vi "Experiment Python Control.vi"() -> ()   [LabVIEW 2015]
uses:
  <vilib>/Platform/TimedLoop/XDataNode/timing_clust.ctl
  <vilib>/Platform/TimedLoop/XDataNode/nitl_modes.ctl
  <vilib>/Platform/TimedLoop/XDataNode/wakeup.ctl
  <vilib>/DAQmx/read.llb/DAQmx Read (Analog 1D DBL NChan 1Samp).vi
  <vilib>/DAQmx/create/channels.llb/DAQmx Create Channel (AI-Voltage-Basic).vi
  <vilib>/Enthought/Python Integration Toolkit/api/Unpack Double.vi
  <vilib>/DAQmx/miscellaneous.llb/DAQmx Fill In Error Info.vi
  <vilib>/Platform/TimedLoop/XDataNode/XDataNode.xnode
  Program Files/neMESYS_SDK/neMESYS LabVIEW Kit/neMESYS LabVIEW Integration Kit.lvlib
  <vilib>/Platform/TimedLoop/XDataNode/XDNodeRunTimeDep.lvlib
  Conor/Temp CN7500/Omega CN7500/Omega CN7500.lvlib
  <vilib>/Enthought/Python Integration Toolkit/Python Integration Toolkit.lvlib
panel:
  out "Desired Conc Not Possible":bool
  out "Boolean 7":bool
  out "Boolean 6":bool
  out "Boolean 5":bool
  out "Boolean 4":bool
  out "Boolean 3":bool
  out "Boolean 2":bool
  out "Boolean 1":bool
  out "Boolean 8":bool
  out "Boolean 0":bool
  out "Flow 8":dbl
  out "Conc 8":dbl
  out "Temp 8":dbl
  out "C BAcid 8":dbl
  out "C EB 8":dbl
  out "Flow 1":dbl
  out "Conc 1":dbl
  out "Temp 1":dbl
  out "C BAcid 1":dbl
  out "C EB 1":dbl
  out "Flow 7":dbl
  out "Conc 7":dbl
  out "Temp 7":dbl
  out "C BAcid 7":dbl
  out "C EB 7":dbl
  out "Flow 6":dbl
  out "Conc 6":dbl
  out "Temp 6":dbl
  out "C BAcid 6":dbl
  out "C EB 6":dbl
  out "Flow 5":dbl
  out "Conc 5":dbl
  out "Temp 5":dbl
  out "C BAcid 5":dbl
  out "C EB 5":dbl
  out "Flow 4":dbl
  out "Conc 4":dbl
  out "Temp 4":dbl
  out "C BAcid 4":dbl
  out "C EB 4":dbl
  out "Flow 3":dbl
  out "Conc 3":dbl
  out "Temp 3":dbl
  out "C BAcid 3":dbl
  out "C EB 3":dbl
  out "Flow 2":dbl
  out "Conc 2":dbl
  out "Temp 2":dbl
  out "C BAcid 2":dbl
  out "C EB 2":dbl
  out "C EB 0":dbl
  out "C BAcid 0":dbl
  out "Temp 0":dbl
  out "Conc 0":dbl
  out "Flow 0":dbl
  in  "Safety or Emergency Syringe Control":bool
  in  "MBDoE or List":bool
  out "Feed Concentration (M)":dbl
  out "Total Flowrate (uL/min)":dbl
  out "Pressure (barg)":dbl
  in  "Shut down in empty?\nLeft off, right on":bool
  out "Text Read From Clipboard 4":string
  out "Read error out 4":errorcluster
  out "Write Set Point Status":string
  out "Error Out 4":i32
  out "Write error out 4":errorcluster
  out "Text Read From Clipboard 3":string
  out "Read error out 3":errorcluster
  out "Read Set Point Status":string
  out "Error Out 3":i32
  out "Write error out 3":errorcluster
  in  "Test Gas Communication":bool
  in  "Change New Set Points":bool
  in  "Read Set Points":bool
  out "Text Read From Clipboard 5":string
  out "Read error out 5":cluster{"source":string}
  out "Write Set Point Status 2":string
  in  "Set Point 1":dbl
  in  "Set Point 2":dbl
  in  "Set Point 3":dbl
  in  "Set Point 4":dbl
  out "Text Read From Clipboard":string
  out "Read error out":errorcluster
  out "Test Status":string
  out "Error Out":i32
  out "Write error out":errorcluster
  out "Text Read From Clipboard 2":string
  out "Read error out 2":errorcluster
  out "Read Flow Status":string
  out "Gas Flow 1":dbl
  out "Gas Flow 2":dbl
  out "Gas Flow 3":dbl
  out "Gas Flow 4":dbl
  out "First waste string":string
  out "Rest of string 1":string
  out "Second Number 2":string
  out "Rest of string 3":string
  out "Third Number 3":string
  out "Rest of string 4":string
  out "Fourth Number 3":string
  out "Rest of string 5":string
  out "Error Out 2":i32
  out "Write error out 2":errorcluster
  in  "Clear":bool
  out "Safety Shut Down Pressure (barg)":dbl
  out "Calculated Pressure":dbl[](graph)
  out "Safety Shut Down Temp":dbl
  out "Actual Temp (oC)":dbl
  out "Temperature":dynamicdata(graph)
  out "Temp Set Point (oC)":dbl
  in  "Temp 8":dbl
  in  "Temp 7":dbl
  in  "Temp 6":dbl
  in  "Temp 5":dbl
  in  "Temp 4":dbl
  in  "Temp 3":dbl
  in  "Temp 2":dbl
  in  "Temp 1":dbl
  in  "Temp 0":dbl
  in  "Update Temperature Set Point":bool
  in  "Automated Experiments or Direct Control":bool
  in  "Set Point (oC)":dbl
  out "loop ind":dbl
  in  "Stop everything":bool
  in  "Skip Exp":bool
  in  "Minutes between Exp":dbl min=0.0 step=0.05
  in  "Refill 4":bool
  in  "Refill 3":bool
  in  "Refill 2":bool
  in  "Refill 1":bool
  in  "Empty 4":bool
  in  "Empty 3":bool
  in  "Empty 2":bool
  in  "Empty 1":bool
  in  "Calibrate 4":bool
  in  "Calibrate 3":bool
  in  "Calibrate 2":bool
  in  "Calibrate 1":bool
  in  "Stop Dose 4":bool
  in  "Stop Dose 3":bool
  in  "Stop Dose 2":bool
  in  "Stop Dose 1":bool
  in  "Flow 8":dbl
  in  "Conc 8":dbl
  in  "Flow 7":dbl
  in  "Conc 7":dbl
  in  "Flow 6":dbl
  in  "Conc 6":dbl
  in  "Flow 5":dbl
  in  "Conc 5":dbl
  in  "Flow 4":dbl
  in  "Conc 4":dbl
  in  "Flow 3":dbl
  in  "Conc 3":dbl
  in  "Flow 2":dbl
  in  "Conc 2":dbl
  in  "Flow 1":dbl
  in  "Conc 1":dbl
  in  "Flow 0":dbl
  in  "Conc 0":dbl
  in  "Generate Flow":bool
  in  "Set Flowrate 1":dbl
  in  "Set Flowrate 2":dbl
  in  "Set Flowrate 3":dbl
  in  "Set Flowrate 4":dbl
  in  "High Conc":dbl min=0.0 max=2.0
  in  "Low Conc":dbl min=0.0 max=2.0
  out "Volumetric Fraction Acid":dbl min=0.0 max=1.0
  out "Syringe Level 4":dbl(slide) scale=0.0..5500.0
  out "Syringe Level 3":dbl(slide) scale=0.0..5500.0
  out "Syringe Level 2":dbl(slide) scale=0.0..5500.0
  out "Syringe Level 1":dbl(slide) scale=0.0..5500.0
  out "Flowrate 4 Ethanol":dbl
  out "Flowrate 3 Acid":dbl
  out "Flowrate 2 Low":dbl
  out "Flowrate 1 High":dbl
  # "Pre Planned Experiments"
  # "Conducted Experiments Set Points"
  # "Current Conditions"
  # "Safety (start and end)"
  # "1 & 2 chosen in advance"
  # "(uL/min)"
  # "3 onwards MBDoE"
  # "Coerced to nearest possible"
  # "Reported Values are set point no actual\nso if set point is not possible\ncoercion takes place\nbut actual is not recorded"
  # "Experimental Info"
  # "Acid must be between 0 and 1, normally 0.1 for 10%"
  # "Direct Control"
  # "Unit of Gas Flow NmL/min"
  # "Emergency Syringe Control Below"
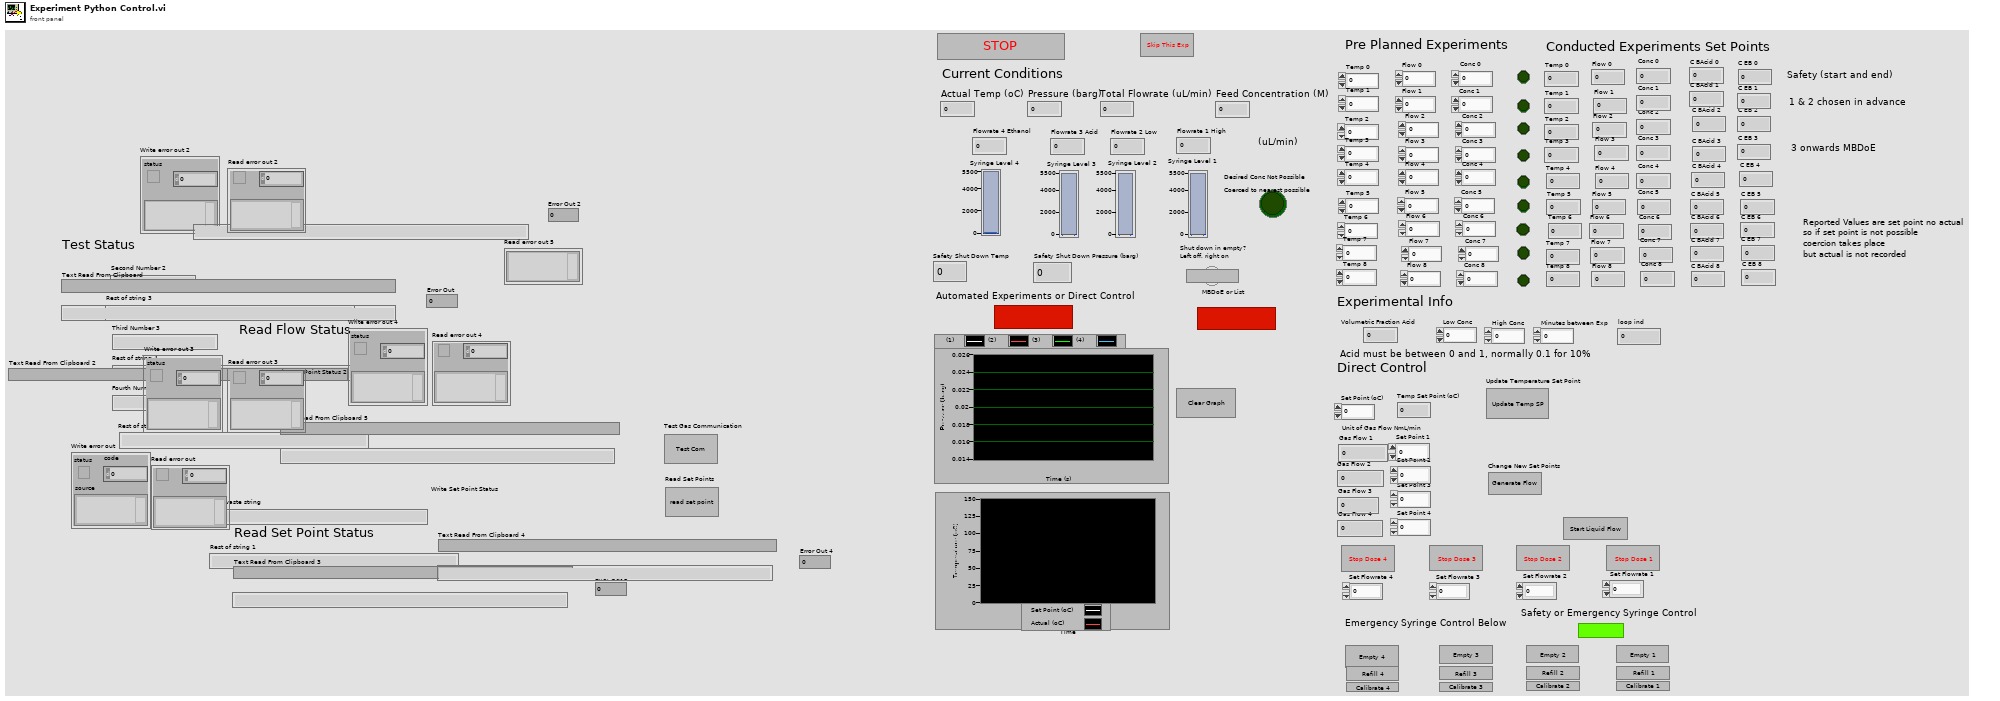
[diagram p1: front panel]
types:
  T1 = typedef "XDNodeRunTimeDep.lvlib/timing_clust.ctl" = cluster{"Expected End [f-1]":u64, "Actual End [f-1]":u64, "Finished Late? [f-1]":bool, "Expected End [i-1]":u64, "Actual End [i-1]":u64, "Finished Late? [i-1]":bool, "Expected Start [i]":u64, "Actual Start [i]":u64, "Expected Start [f]":u64, "Actual Start [f]":u64, "Source Name":string, "Structure Name":string, "Period":i64, "Deadline":i64, "Offset":i64, "Start":i64, "Priority":i32, "Timeout":i32, "Mode":T2, "Wakeup Reason":T3, "Error":errorcluster, "Source Type":string, "Secondary Source Type":string, "Global End Time":u64, "Global Start Time":u64, "Frame Duration":u64, "Iteration Duration":u64, "Assigned CPU":i32, "I/O Scan Engine Mode":u32}
  T2 = typedef "XDNodeRunTimeDep.lvlib/nitl_modes.ctl" = enum32{"No Change", "Process missed periods, maintain original phase", "Discard missed periods, maintain original phase", "Process missed periods, ignore original phase", "Discard missed periods, ignore original phase"}
  T3 = typedef "XDNodeRunTimeDep.lvlib/wakeup.ctl" = enum32{"Normal", "Aborted", "Asynchronous wakeup", "Timing source error", "Timed loop error", "Timeout"}
  T4 = typedef "Python Integration Toolkit.lvlib/Session ID.ctl" = u64
  T5 = typedef "Python Integration Toolkit.lvlib/Python Objects.ctl" = variant
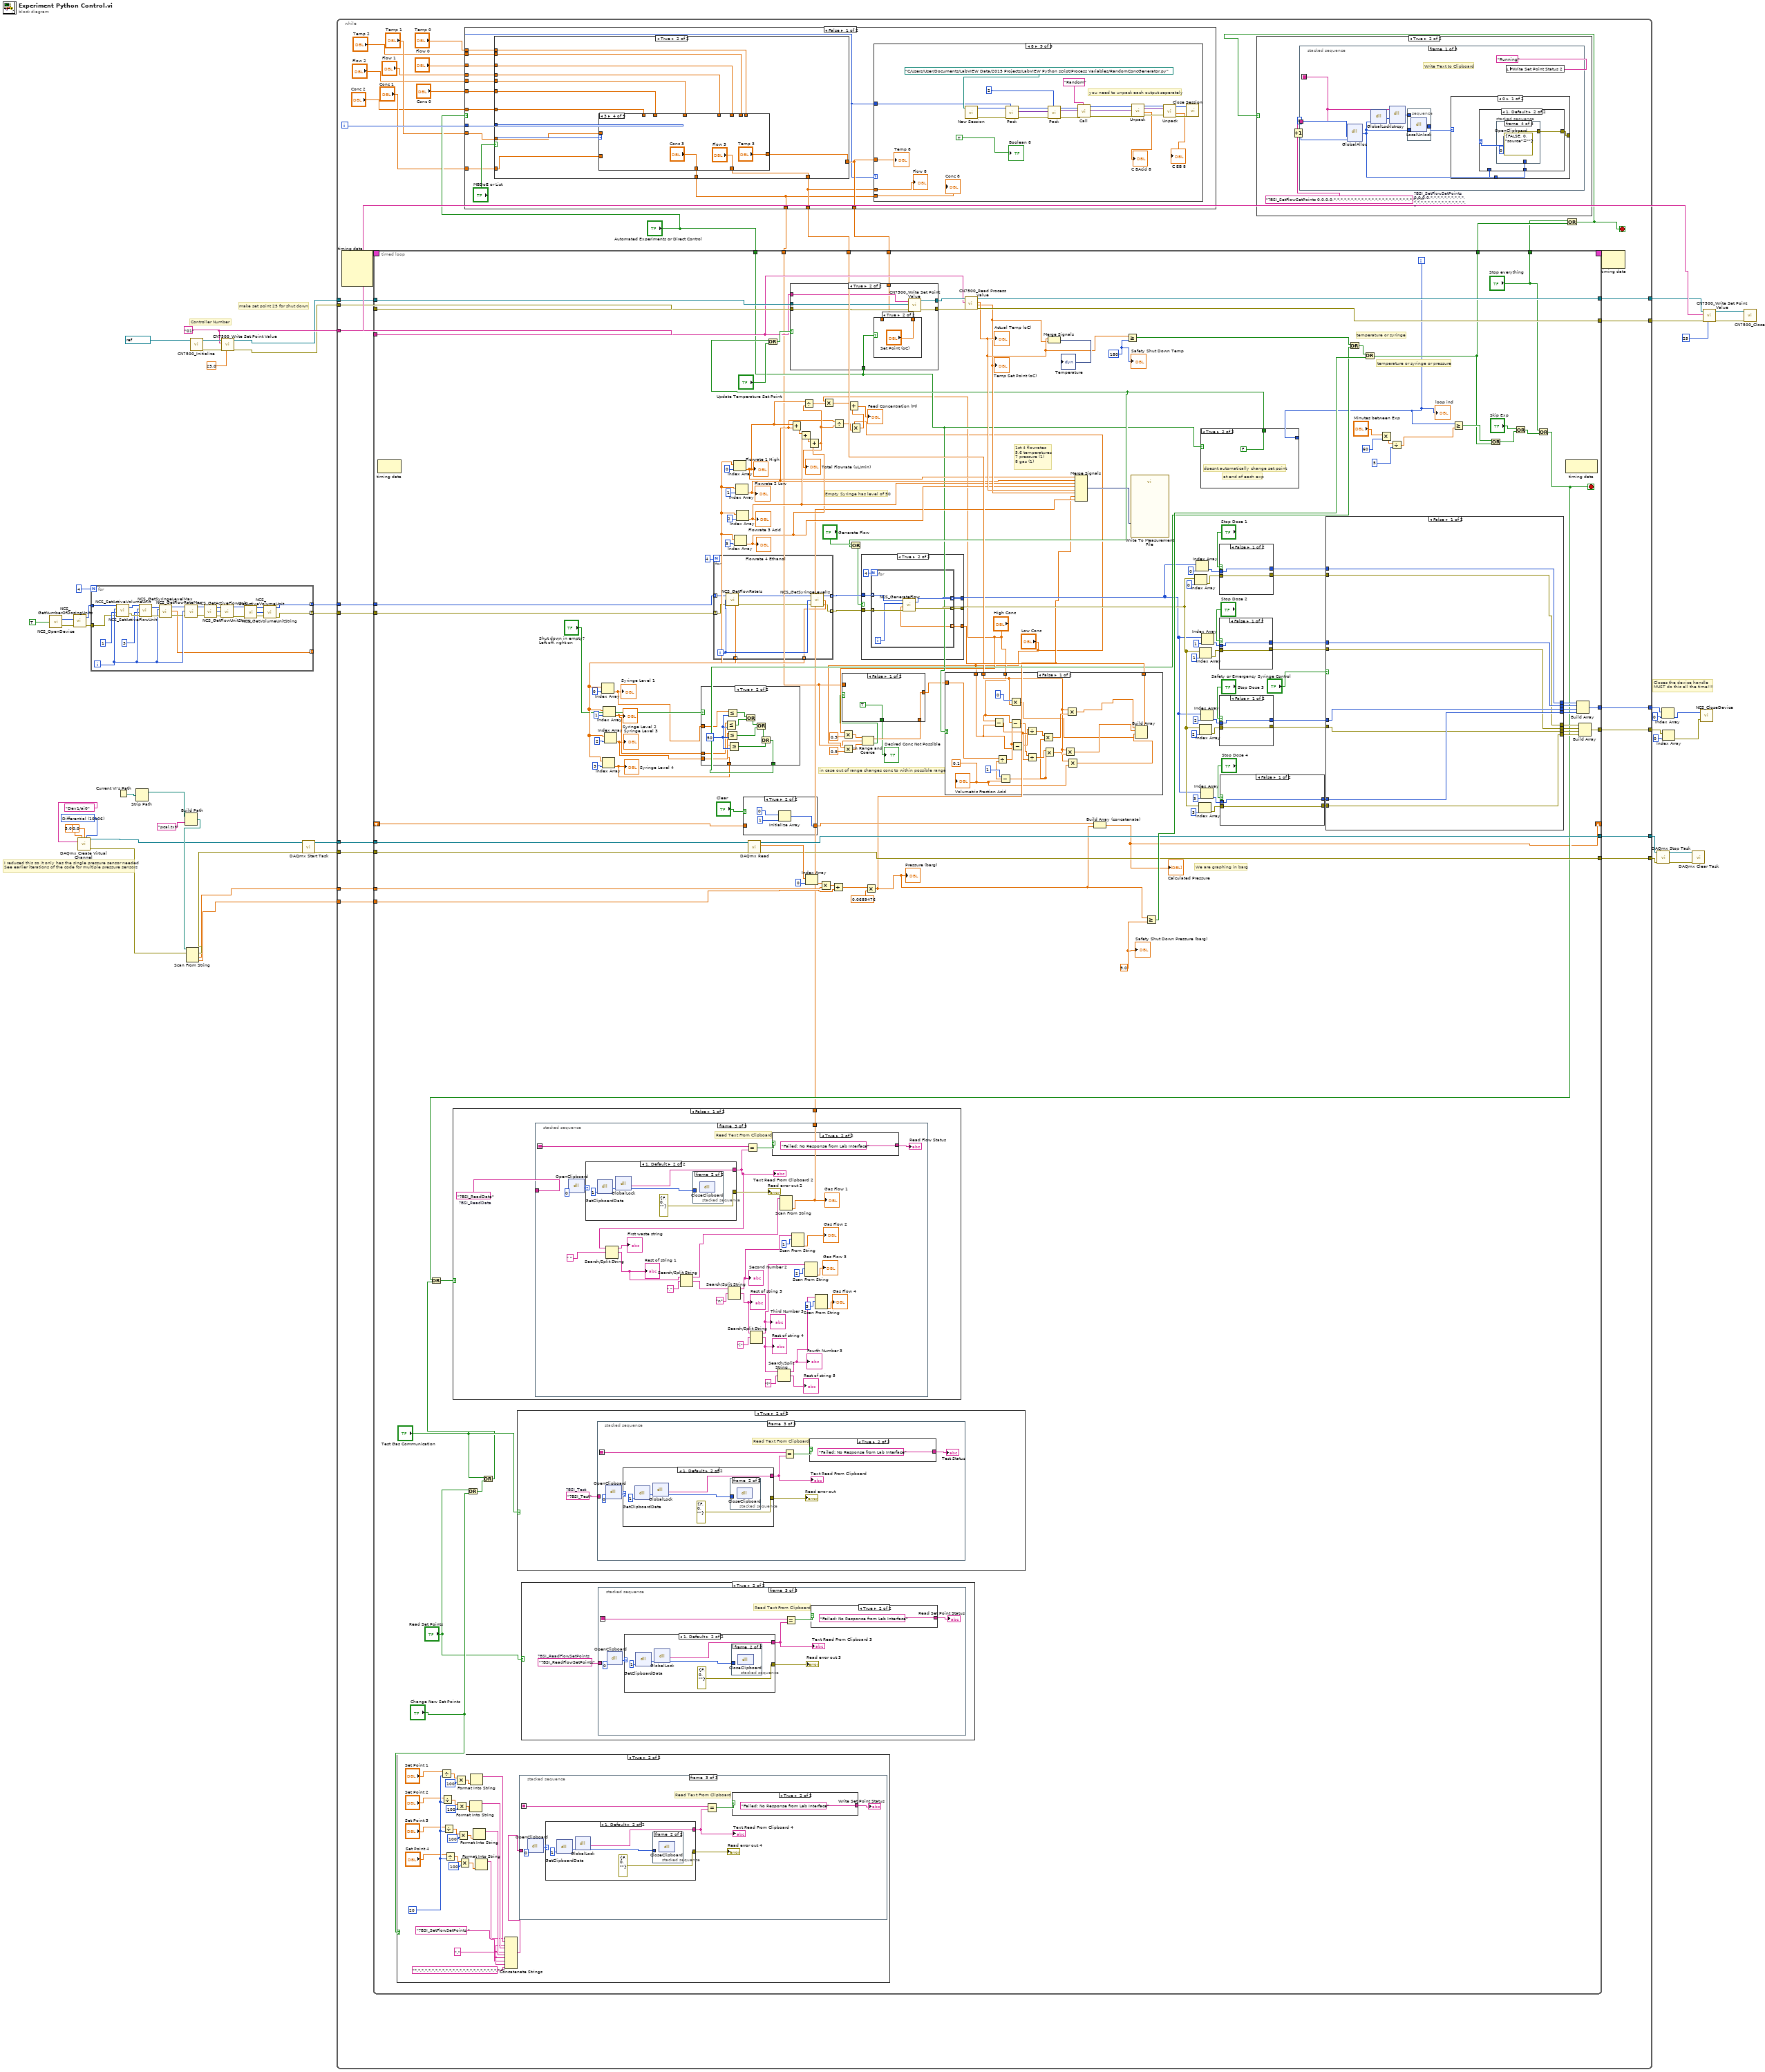
[diagram p0: block diagram]
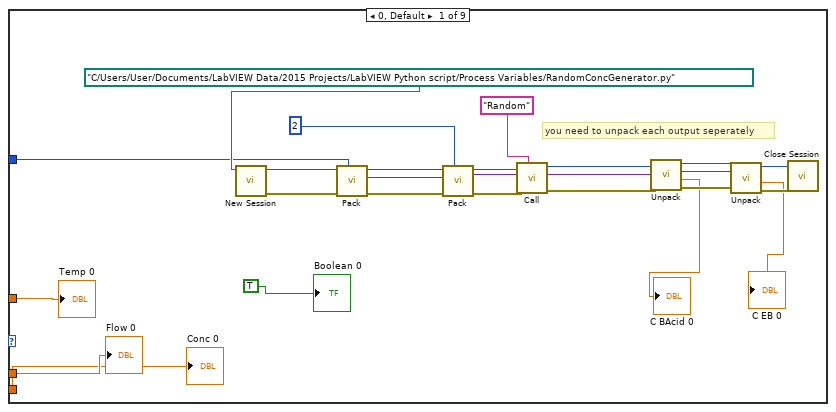
[diagram p2: hidden frame]
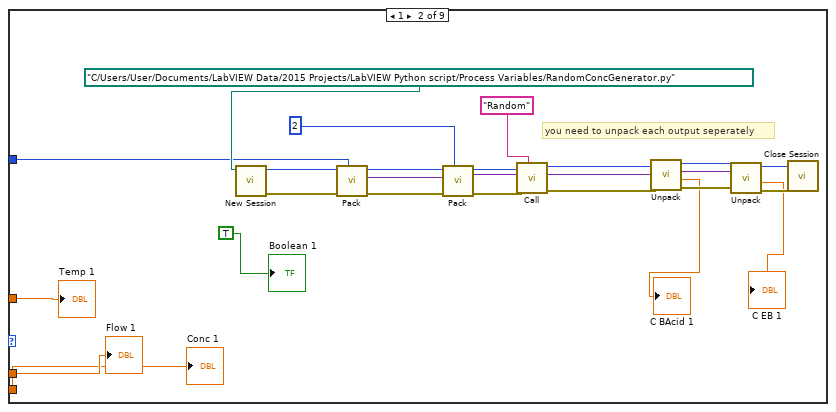
[diagram p3: hidden frame]
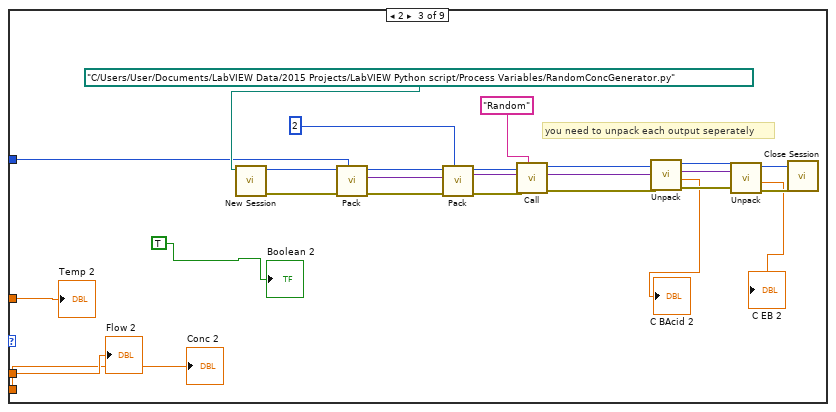
[diagram p4: hidden frame]
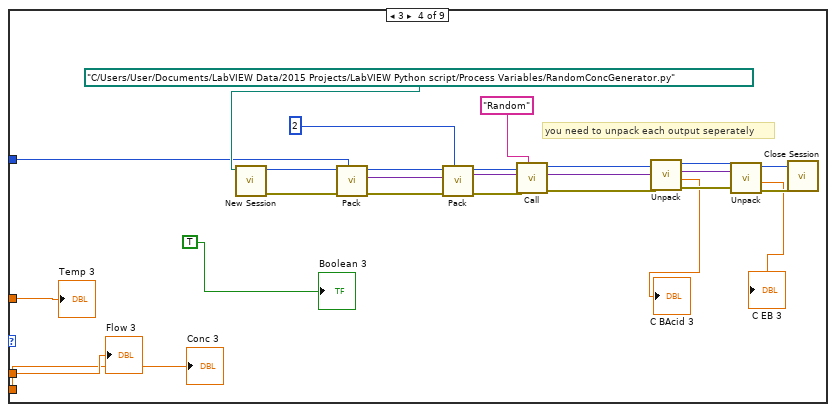
[diagram p5: hidden frame]
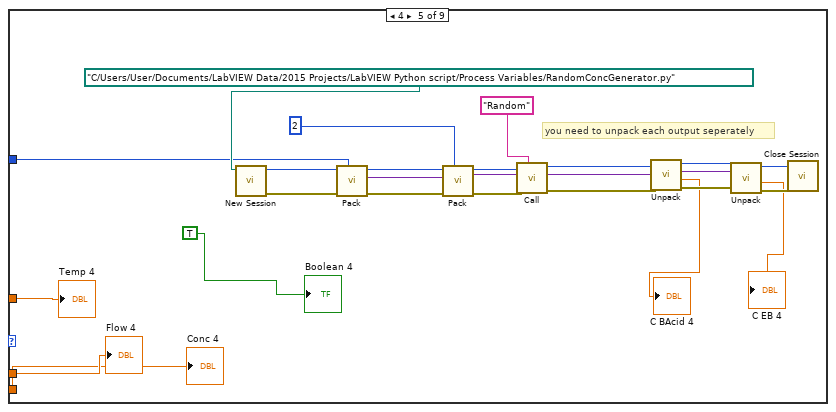
[diagram p6: hidden frame]
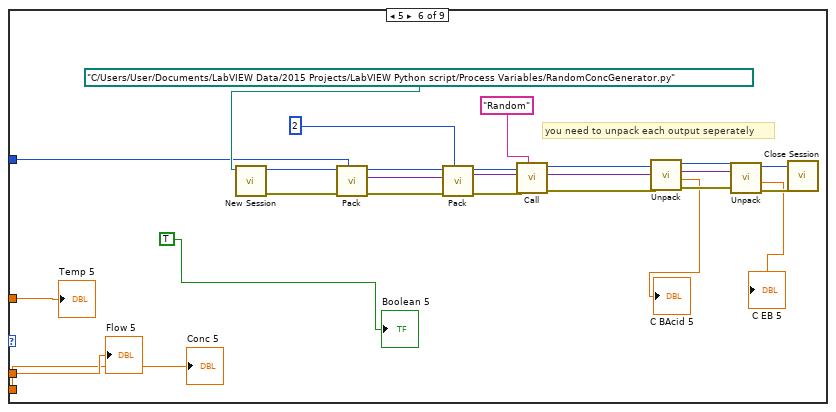
[diagram p7: hidden frame]
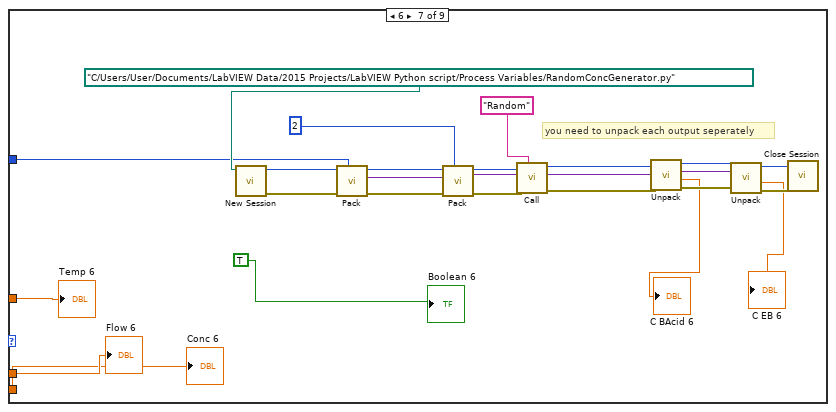
[diagram p8: hidden frame]
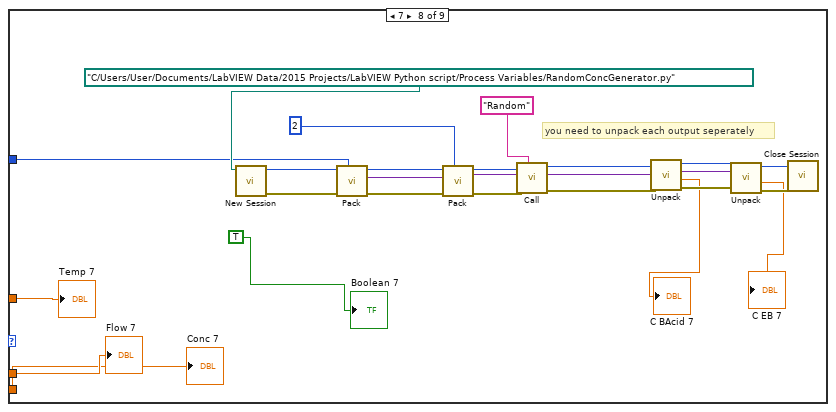
[diagram p9: hidden frame]
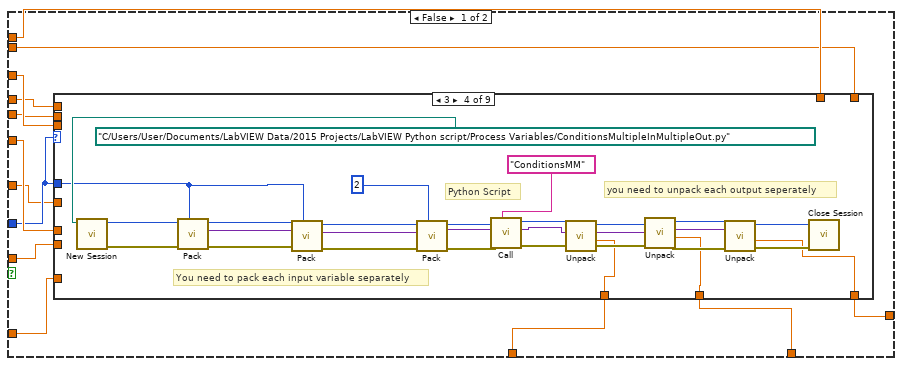
[diagram p10: hidden frame]
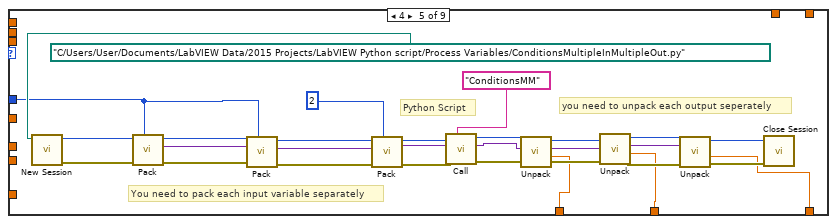
[diagram p14: hidden frame]
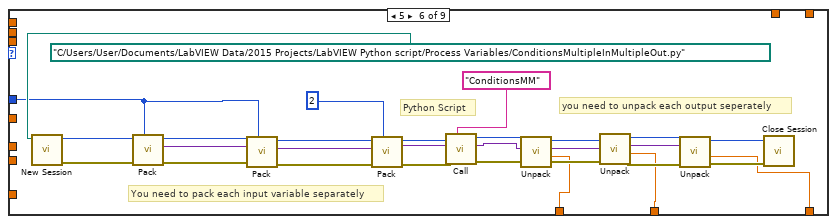
[diagram p15: hidden frame]
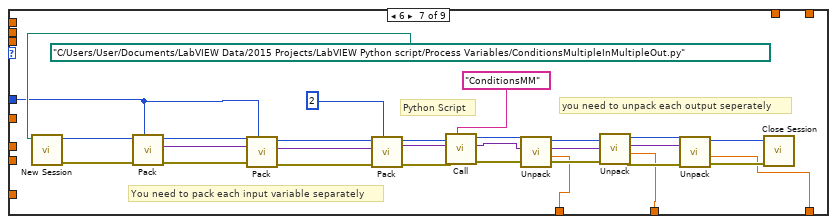
[diagram p16: hidden frame]
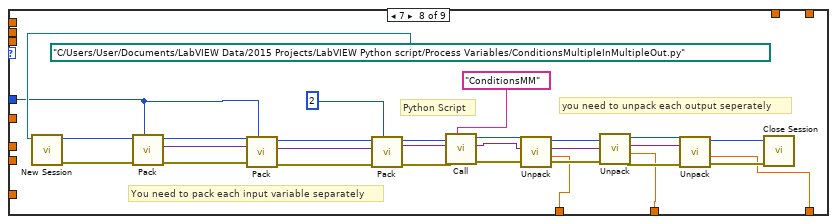
[diagram p17: hidden frame]
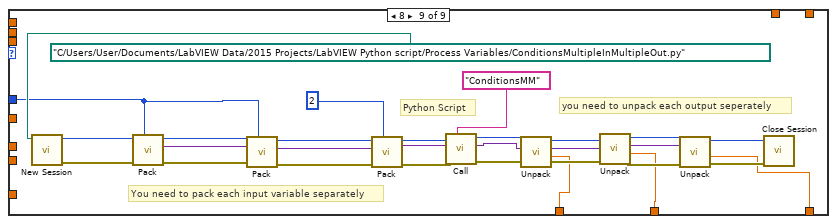
[diagram p18: hidden frame]
diagram:
  w17 = 10106 items=["default"=-1, "RSE"=10083, "NRSE"=10078, "Differential"=10106, "Pseudodifferential"=12529] ("input terminal configuration")
  w24 = "01" ("Controller Number")
  # "I reduced this so it only has the single pressure sensor needed\nSee earlier iterations of the code for multiple pressure sensors"
  # "make set point 25 for shut down"
  # "Controller Number"
  # "Closes the device handle \nMUST do this all the time!!!!"
  n1 = call "NCS_OpenDevice.vi"("show status window"=TRUE) -> ("device handle"=w43:u32, "error out"=w42:errorcluster)
  n2 = call "NCS_GetNumberOfDosingUnits.vi"("device handle in"=w43, "error in (no error)"=w42) -> ("device handle out"=w40:u32, "error out"=w41:errorcluster)  [unwired: 1 out]
  n3 = call-poly <vilib>:"DAQmx Create Virtual Channel.vi"("maximum value"=5.0, "minimum value"=0.0, "input terminal configuration"=w17, "physical channels"=tag "Dev1/ai0") -> ("task out"=w1:refnum<k21>, "error out"=w2:errorcluster)  [unwired: 10 in]
  n4 = for {
    N: 4 -> [_]
    tunnel: [w49] -> w39 mode=indexing
    tunnel: [w48] -> w38 mode=indexing
    tunnel: [w62] -> _ mode=indexing
    tunnel: w41 -> [w47]
    tunnel: w40 -> [w46]
    i -> [w65]
    n5 = call "NCS_SetActiveVolumeUnit.vi"("error in (no error)"=w47, "active volume unit"=1, "dosingunit"=w65, "device handle in"=w46) -> ("error out"=w68:errorcluster, "device handle out"=w69:u32)
    n6 = call "NCS_SetActiveFlowUnit.vi"("error in (no error)"=w68, "active flow unit"=3, "dosingunit"=w65, "device handle in"=w69) -> ("error out"=w66:errorcluster, "device handle out"=w67:u32)
    n7 = call "NCS_GetSyringeLevelMax.vi"("error in (no error)"=w66, "dosingunit"=w65, "device handle in"=w67) -> ("error out"=w63:errorcluster, "syringe level max"=w62:dbl, "device handle out"=w64:u32)  [unwired: 1 out]
    n8 = call "NCS_GetFlowRateMax.vi"("error in (no error)"=w63, "dosingunit"=w65, "device handle in"=w64) -> ("error out"=w50:errorcluster, "device handle out"=w51:u32)  [unwired: 1 out]
    n9 = call "NCS_GetActiveFlowUnit.vi"("error in (no error)"=w50, "device handle in"=w51) -> ("error out"=w58:errorcluster, "active flow unit"=w57:u8, "device handle out"=w59:u32)  [unwired: 1 in]
    n10 = call "NCS_GetFlowUnitString.vi"("device handle in"=w59, "flow unit id"=w57, "error in (no error)"=w58) -> ("device handle out"=w54:u32, "error out"=w53:errorcluster)  [unwired: 2 out]
    n11 = call "NCS_GetActiveVolumeUnit.vi"("error in (no error)"=w53, "device handle in"=w54) -> ("error out"=w55:errorcluster, "active volume unit"=w56:u8, "device handle out"=w52:u32)  [unwired: 1 in]
    n12 = call "NCS_GetVolumeUnitString.vi"("device handle in"=w52, "volume unit id"=w56, "error in (no error)"=w55) -> ("device handle out"=w49:u32, "error out"=w48:errorcluster)  [unwired: 2 out]
  }
  n13 = Current VI's Path() -> (path=w15:path)
  n14 = Strip Path(path=w15) -> (stripped path=w13:path)  [unwired: 1 out]
  n15 = Build Path(base path=w13, name or relative path="pcal.txt") -> (appended path=w14:path)
  n16 = Scan From String(w14, w2) -> (w11:errorcluster, output 1=w8:dbl, output 2=w7:dbl)  [unwired: 3 in, 1 out]
  n17 = call "CN7500_Initialize.vi"("VISA resource name"=refnum<visa-resource-name> "COM8") -> ("error out"=w30:errorcluster, "VISA resource name out"=w31:refnum<visa-resource-name>)  [unwired: 9 in]
  n18 = call "CN7500_Write Set Point Value.vi"("Target Set Point Value"=25.0, "error in (no error)"=w30, "Controller Number"=w24, "VISA In"=w31) -> ("error out"=w22:errorcluster, "VISA Out"=w23:refnum<visa-resource-name>)  [unwired: 6 in]
  n19 = call <vilib>:"DAQmx Start Task.vi"("task/channels in"=w1, "error in"=w11) -> ("task out"=w10:refnum<k21>, "error out"=w9:errorcluster)  [unwired: 12 in]
  n20 = while {
    tunnel: w39 -> [w103]
    tunnel: w38 -> [w102]
    tunnel: [w101] -> w33
    tunnel: [w100] -> w32
    tunnel: w24 -> [w97]
    tunnel: w23 -> [w96]
    tunnel: w22 -> [w95]
    tunnel: [w94] -> w21
    tunnel: [w93] -> w20
    tunnel: w10 -> [w91]
    tunnel: w9 -> [w90]
    tunnel: w8 -> [w89]
    tunnel: w7 -> [w88]
    tunnel: [w87] -> w4
    tunnel: [w86] -> w3
    i -> [w80]
    stop <- w85 stop-if-true
    n21 = node-c288() -> (w99:T1)  [unwired: 4 in]
    n22 = case shown="False" "Automated Experiments or Direct Control" {
      tunnel: [w116 w588] -> w83
      tunnel: [w115 w588] -> w82
      tunnel: [w114 w588] -> w81
      tunnel: w80 -> [w113 _]
      tunnel: "Conc 0" -> [w112 _]
      tunnel: "Flow 0" -> [w111 _]
      tunnel: "Temp 0" -> [w110 _]
      tunnel: "Temp 1" -> [w109 _]
      tunnel: "Flow 1" -> [w108 _]
      tunnel: "Conc 1" -> [w107 _]
      tunnel: "Temp 2" -> [w106 _]
      tunnel: "Flow 2" -> [w105 _]
      tunnel: "Conc 2" -> [w104 _]
      frame False {
        n23 = case shown="True" "MBDoE or List" {
          tunnel: [w362 w560] -> w116
          tunnel: [w363 w559] -> w115
          tunnel: [w364 w558] -> w114
          tunnel: w113 -> [w358 w557]
          tunnel: w112 -> [w361 w556]
          tunnel: w111 -> [w360 w555]
          tunnel: w110 -> [w359 w554]
          tunnel: w109 -> [w357 w553]
          tunnel: w108 -> [w356 w552]
          tunnel: w107 -> [w355 w551]
          tunnel: w106 -> [w354 w550]
          tunnel: w105 -> [w353 w549]
          tunnel: w104 -> [w352 w548]
          frame False {
            n24 = case shown="3" w358 {
              tunnel: w358 -> [_ _ _ w378 w407 w436 w465 w494 w523]
              tunnel: [w367 w368 w371 w376 w405 w434 w463 w492 w521] -> w364
              tunnel: [w366 w369 w372 w375 w404 w433 w462 w491 w520] -> w363
              tunnel: [w365 w370 w373 w374 w403 w432 w461 w490 w519] -> w362
              tunnel: w361 -> [w367 _ _ _ _ _ _ _ _]
              tunnel: w360 -> [w366 _ _ _ _ _ _ _ _]
              tunnel: w359 -> [w365 _ _ _ _ _ _ _ _]
              tunnel: w357 -> [_ w370 _ _ _ _ _ _ _]
              tunnel: w356 -> [_ w369 _ _ _ _ _ _ _]
              tunnel: w355 -> [_ w368 _ _ _ _ _ _ _]
              tunnel: w354 -> [_ _ w373 _ _ _ _ _ _]
              tunnel: w353 -> [_ _ w372 _ _ _ _ _ _]
              tunnel: w352 -> [_ _ w371 _ _ _ _ _ _]
              frame 0, Default {
                # "start and end safety"
              }
              frame 1 {
              }
              frame 2 {
              }
              frame 3 {
                # "you need to unpack each output seperately"
                # "You need to pack each input variable separately"
                # "Python Script"
                n25 = call <vilib>:"New Session.vi"("Path to Python Module (.py File)"=path "C:/Users/User/Documents/LabVIEW Data/2015 Projects/LabVIEW Python script/Process Variables/ConditionsMultipleInMultipleOut.py") -> ("error out"=w391:errorcluster, "Session ID out"=w394:T4)  [unwired: 9 in]
                n26 = call <vilib>:"Pack.vi"("Argument"=w378, "error in (no error)"=w391, "Session ID"=w394) -> ("error out"=w390:errorcluster, "Python Object References Out"=w388:T5, "Session ID out"=w393:T4)  [unwired: 6 in]
                n27 = call <vilib>:"Pack.vi"("Argument"=w378, "error in (no error)"=w390, "Python Object References In"=w388, "Session ID"=w393) -> ("error out"=w389:errorcluster, "Python Object References Out"=w387:T5, "Session ID out"=w392:T4)  [unwired: 5 in]
                n28 = call <vilib>:"Pack.vi"("Argument"=2, "error in (no error)"=w389, "Python Object References In"=w387, "Session ID"=w392) -> ("error out"=w398:errorcluster, "Python Object References Out"=w397:T5, "Session ID out"=w399:T4)  [unwired: 5 in]
                n29 = call <vilib>:"Call.vi"("Function or Method Name"="ConditionsMM", "error in (no error)"=w398, "Python Object References In"=w397, "Session ID"=w399) -> ("error out"=w402:errorcluster, "Python Object References Out"=w401:T5, "Session ID out"=w400:T4)  [unwired: 5 in]
                n30 = call-poly <vilib>:"Unpack.vi"("error in (no error)"=w402, "Python Object References In"=w401, "Session ID"=w400) -> ("error out"=w381:errorcluster, "Value"=w376:dbl, "Python Object References Out"=w380:T5, "Session ID out"=w386:T4)  [unwired: 5 in]
                n31 = call-poly <vilib>:"Unpack.vi"("error in (no error)"=w381, "Python Object References In"=w380, "Session ID"=w386) -> ("error out"=w382:errorcluster, "Value"=w375:dbl, "Python Object References Out"=w379:T5, "Session ID out"=w385:T4)  [unwired: 5 in]
                n32 = call-poly <vilib>:"Unpack.vi"("error in (no error)"=w382, "Python Object References In"=w379, "Session ID"=w385) -> ("error out"=w383:errorcluster, "Value"=w374:dbl, "Session ID out"=w384:T4)  [unwired: 5 in, 1 out]
                n33 = call <vilib>:"Close Session.vi"("error in (no error)"=w383, "Session ID"=w384) -> ()  [unwired: 9 in, 1 out]
              }
              frame 4 {
                # "you need to unpack each output seperately"
                # "You need to pack each input variable separately"
                # "Python Script"
                n34 = call <vilib>:"New Session.vi"("Path to Python Module (.py File)"=path "C:/Users/User/Documents/LabVIEW Data/2015 Projects/LabVIEW Python script/Process Variables/ConditionsMultipleInMultipleOut.py") -> ("error out"=w420:errorcluster, "Session ID out"=w423:T4)  [unwired: 9 in]
                n35 = call <vilib>:"Pack.vi"("Argument"=w407, "error in (no error)"=w420, "Session ID"=w423) -> ("error out"=w419:errorcluster, "Python Object References Out"=w417:T5, "Session ID out"=w422:T4)  [unwired: 6 in]
                n36 = call <vilib>:"Pack.vi"("Argument"=w407, "error in (no error)"=w419, "Python Object References In"=w417, "Session ID"=w422) -> ("error out"=w418:errorcluster, "Python Object References Out"=w416:T5, "Session ID out"=w421:T4)  [unwired: 5 in]
                n37 = call <vilib>:"Pack.vi"("Argument"=2, "error in (no error)"=w418, "Python Object References In"=w416, "Session ID"=w421) -> ("error out"=w427:errorcluster, "Python Object References Out"=w426:T5, "Session ID out"=w428:T4)  [unwired: 5 in]
                n38 = call <vilib>:"Call.vi"("Function or Method Name"="ConditionsMM", "error in (no error)"=w427, "Python Object References In"=w426, "Session ID"=w428) -> ("error out"=w431:errorcluster, "Python Object References Out"=w430:T5, "Session ID out"=w429:T4)  [unwired: 5 in]
                n39 = call-poly <vilib>:"Unpack.vi"("error in (no error)"=w431, "Python Object References In"=w430, "Session ID"=w429) -> ("error out"=w410:errorcluster, "Value"=w405:dbl, "Python Object References Out"=w409:T5, "Session ID out"=w415:T4)  [unwired: 5 in]
                n40 = call-poly <vilib>:"Unpack.vi"("error in (no error)"=w410, "Python Object References In"=w409, "Session ID"=w415) -> ("error out"=w411:errorcluster, "Value"=w404:dbl, "Python Object References Out"=w408:T5, "Session ID out"=w414:T4)  [unwired: 5 in]
                n41 = call-poly <vilib>:"Unpack.vi"("error in (no error)"=w411, "Python Object References In"=w408, "Session ID"=w414) -> ("error out"=w412:errorcluster, "Value"=w403:dbl, "Session ID out"=w413:T4)  [unwired: 5 in, 1 out]
                n42 = call <vilib>:"Close Session.vi"("error in (no error)"=w412, "Session ID"=w413) -> ()  [unwired: 9 in, 1 out]
              }
              frame 5 {
                # "you need to unpack each output seperately"
                # "You need to pack each input variable separately"
                # "Python Script"
                n43 = call <vilib>:"New Session.vi"("Path to Python Module (.py File)"=path "C:/Users/User/Documents/LabVIEW Data/2015 Projects/LabVIEW Python script/Process Variables/ConditionsMultipleInMultipleOut.py") -> ("error out"=w449:errorcluster, "Session ID out"=w452:T4)  [unwired: 9 in]
                n44 = call <vilib>:"Pack.vi"("Argument"=w436, "error in (no error)"=w449, "Session ID"=w452) -> ("error out"=w448:errorcluster, "Python Object References Out"=w446:T5, "Session ID out"=w451:T4)  [unwired: 6 in]
                n45 = call <vilib>:"Pack.vi"("Argument"=w436, "error in (no error)"=w448, "Python Object References In"=w446, "Session ID"=w451) -> ("error out"=w447:errorcluster, "Python Object References Out"=w445:T5, "Session ID out"=w450:T4)  [unwired: 5 in]
                n46 = call <vilib>:"Pack.vi"("Argument"=2, "error in (no error)"=w447, "Python Object References In"=w445, "Session ID"=w450) -> ("error out"=w456:errorcluster, "Python Object References Out"=w455:T5, "Session ID out"=w457:T4)  [unwired: 5 in]
                n47 = call <vilib>:"Call.vi"("Function or Method Name"="ConditionsMM", "error in (no error)"=w456, "Python Object References In"=w455, "Session ID"=w457) -> ("error out"=w460:errorcluster, "Python Object References Out"=w459:T5, "Session ID out"=w458:T4)  [unwired: 5 in]
                n48 = call-poly <vilib>:"Unpack.vi"("error in (no error)"=w460, "Python Object References In"=w459, "Session ID"=w458) -> ("error out"=w439:errorcluster, "Value"=w434:dbl, "Python Object References Out"=w438:T5, "Session ID out"=w444:T4)  [unwired: 5 in]
                n49 = call-poly <vilib>:"Unpack.vi"("error in (no error)"=w439, "Python Object References In"=w438, "Session ID"=w444) -> ("error out"=w440:errorcluster, "Value"=w433:dbl, "Python Object References Out"=w437:T5, "Session ID out"=w443:T4)  [unwired: 5 in]
                n50 = call-poly <vilib>:"Unpack.vi"("error in (no error)"=w440, "Python Object References In"=w437, "Session ID"=w443) -> ("error out"=w441:errorcluster, "Value"=w432:dbl, "Session ID out"=w442:T4)  [unwired: 5 in, 1 out]
                n51 = call <vilib>:"Close Session.vi"("error in (no error)"=w441, "Session ID"=w442) -> ()  [unwired: 9 in, 1 out]
              }
              frame 6 {
                # "you need to unpack each output seperately"
                # "You need to pack each input variable separately"
                # "Python Script"
                n52 = call <vilib>:"New Session.vi"("Path to Python Module (.py File)"=path "C:/Users/User/Documents/LabVIEW Data/2015 Projects/LabVIEW Python script/Process Variables/ConditionsMultipleInMultipleOut.py") -> ("error out"=w478:errorcluster, "Session ID out"=w481:T4)  [unwired: 9 in]
                n53 = call <vilib>:"Pack.vi"("Argument"=w465, "error in (no error)"=w478, "Session ID"=w481) -> ("error out"=w477:errorcluster, "Python Object References Out"=w475:T5, "Session ID out"=w480:T4)  [unwired: 6 in]
                n54 = call <vilib>:"Pack.vi"("Argument"=w465, "error in (no error)"=w477, "Python Object References In"=w475, "Session ID"=w480) -> ("error out"=w476:errorcluster, "Python Object References Out"=w474:T5, "Session ID out"=w479:T4)  [unwired: 5 in]
                n55 = call <vilib>:"Pack.vi"("Argument"=2, "error in (no error)"=w476, "Python Object References In"=w474, "Session ID"=w479) -> ("error out"=w485:errorcluster, "Python Object References Out"=w484:T5, "Session ID out"=w486:T4)  [unwired: 5 in]
                n56 = call <vilib>:"Call.vi"("Function or Method Name"="ConditionsMM", "error in (no error)"=w485, "Python Object References In"=w484, "Session ID"=w486) -> ("error out"=w489:errorcluster, "Python Object References Out"=w488:T5, "Session ID out"=w487:T4)  [unwired: 5 in]
                n57 = call-poly <vilib>:"Unpack.vi"("error in (no error)"=w489, "Python Object References In"=w488, "Session ID"=w487) -> ("error out"=w468:errorcluster, "Value"=w463:dbl, "Python Object References Out"=w467:T5, "Session ID out"=w473:T4)  [unwired: 5 in]
                n58 = call-poly <vilib>:"Unpack.vi"("error in (no error)"=w468, "Python Object References In"=w467, "Session ID"=w473) -> ("error out"=w469:errorcluster, "Value"=w462:dbl, "Python Object References Out"=w466:T5, "Session ID out"=w472:T4)  [unwired: 5 in]
                n59 = call-poly <vilib>:"Unpack.vi"("error in (no error)"=w469, "Python Object References In"=w466, "Session ID"=w472) -> ("error out"=w470:errorcluster, "Value"=w461:dbl, "Session ID out"=w471:T4)  [unwired: 5 in, 1 out]
                n60 = call <vilib>:"Close Session.vi"("error in (no error)"=w470, "Session ID"=w471) -> ()  [unwired: 9 in, 1 out]
              }
              frame 7 {
                # "you need to unpack each output seperately"
                # "You need to pack each input variable separately"
                # "Python Script"
                n61 = call <vilib>:"New Session.vi"("Path to Python Module (.py File)"=path "C:/Users/User/Documents/LabVIEW Data/2015 Projects/LabVIEW Python script/Process Variables/ConditionsMultipleInMultipleOut.py") -> ("error out"=w507:errorcluster, "Session ID out"=w510:T4)  [unwired: 9 in]
                n62 = call <vilib>:"Pack.vi"("Argument"=w494, "error in (no error)"=w507, "Session ID"=w510) -> ("error out"=w506:errorcluster, "Python Object References Out"=w504:T5, "Session ID out"=w509:T4)  [unwired: 6 in]
                n63 = call <vilib>:"Pack.vi"("Argument"=w494, "error in (no error)"=w506, "Python Object References In"=w504, "Session ID"=w509) -> ("error out"=w505:errorcluster, "Python Object References Out"=w503:T5, "Session ID out"=w508:T4)  [unwired: 5 in]
                n64 = call <vilib>:"Pack.vi"("Argument"=2, "error in (no error)"=w505, "Python Object References In"=w503, "Session ID"=w508) -> ("error out"=w514:errorcluster, "Python Object References Out"=w513:T5, "Session ID out"=w515:T4)  [unwired: 5 in]
                n65 = call <vilib>:"Call.vi"("Function or Method Name"="ConditionsMM", "error in (no error)"=w514, "Python Object References In"=w513, "Session ID"=w515) -> ("error out"=w518:errorcluster, "Python Object References Out"=w517:T5, "Session ID out"=w516:T4)  [unwired: 5 in]
                n66 = call-poly <vilib>:"Unpack.vi"("error in (no error)"=w518, "Python Object References In"=w517, "Session ID"=w516) -> ("error out"=w497:errorcluster, "Value"=w492:dbl, "Python Object References Out"=w496:T5, "Session ID out"=w502:T4)  [unwired: 5 in]
                n67 = call-poly <vilib>:"Unpack.vi"("error in (no error)"=w497, "Python Object References In"=w496, "Session ID"=w502) -> ("error out"=w498:errorcluster, "Value"=w491:dbl, "Python Object References Out"=w495:T5, "Session ID out"=w501:T4)  [unwired: 5 in]
                n68 = call-poly <vilib>:"Unpack.vi"("error in (no error)"=w498, "Python Object References In"=w495, "Session ID"=w501) -> ("error out"=w499:errorcluster, "Value"=w490:dbl, "Session ID out"=w500:T4)  [unwired: 5 in, 1 out]
                n69 = call <vilib>:"Close Session.vi"("error in (no error)"=w499, "Session ID"=w500) -> ()  [unwired: 9 in, 1 out]
              }
              frame 8 {
                # "you need to unpack each output seperately"
                # "You need to pack each input variable separately"
                # "Python Script"
                n70 = call <vilib>:"New Session.vi"("Path to Python Module (.py File)"=path "C:/Users/User/Documents/LabVIEW Data/2015 Projects/LabVIEW Python script/Process Variables/ConditionsMultipleInMultipleOut.py") -> ("error out"=w536:errorcluster, "Session ID out"=w539:T4)  [unwired: 9 in]
                n71 = call <vilib>:"Pack.vi"("Argument"=w523, "error in (no error)"=w536, "Session ID"=w539) -> ("error out"=w535:errorcluster, "Python Object References Out"=w533:T5, "Session ID out"=w538:T4)  [unwired: 6 in]
                n72 = call <vilib>:"Pack.vi"("Argument"=w523, "error in (no error)"=w535, "Python Object References In"=w533, "Session ID"=w538) -> ("error out"=w534:errorcluster, "Python Object References Out"=w532:T5, "Session ID out"=w537:T4)  [unwired: 5 in]
                n73 = call <vilib>:"Pack.vi"("Argument"=2, "error in (no error)"=w534, "Python Object References In"=w532, "Session ID"=w537) -> ("error out"=w543:errorcluster, "Python Object References Out"=w542:T5, "Session ID out"=w544:T4)  [unwired: 5 in]
                n74 = call <vilib>:"Call.vi"("Function or Method Name"="ConditionsMM", "error in (no error)"=w543, "Python Object References In"=w542, "Session ID"=w544) -> ("error out"=w547:errorcluster, "Python Object References Out"=w546:T5, "Session ID out"=w545:T4)  [unwired: 5 in]
                n75 = call-poly <vilib>:"Unpack.vi"("error in (no error)"=w547, "Python Object References In"=w546, "Session ID"=w545) -> ("error out"=w526:errorcluster, "Value"=w521:dbl, "Python Object References Out"=w525:T5, "Session ID out"=w531:T4)  [unwired: 5 in]
                n76 = call-poly <vilib>:"Unpack.vi"("error in (no error)"=w526, "Python Object References In"=w525, "Session ID"=w531) -> ("error out"=w527:errorcluster, "Value"=w520:dbl, "Python Object References Out"=w524:T5, "Session ID out"=w530:T4)  [unwired: 5 in]
                n77 = call-poly <vilib>:"Unpack.vi"("error in (no error)"=w527, "Python Object References In"=w524, "Session ID"=w530) -> ("error out"=w528:errorcluster, "Value"=w519:dbl, "Session ID out"=w529:T4)  [unwired: 5 in, 1 out]
                n78 = call <vilib>:"Close Session.vi"("error in (no error)"=w528, "Session ID"=w529) -> ()  [unwired: 9 in, 1 out]
              }
            }
          }
          frame True {
            n79 = case shown="3" w557 {
              tunnel: [w562 w565 w568 "Flow 3" "Flow 4" "Flow 5" "Flow 6" "Flow 7" "Flow 8"] -> w559
              tunnel: [w563 w564 w567 "Conc 3" "Conc 4" "Conc 5" "Conc 6" "Conc 7" "Conc 8"] -> w558
              tunnel: [w561 w566 w569 "Temp 3" "Temp 4" "Temp 5" "Temp 6" "Temp 7" "Temp 8"] -> w560
              tunnel: w556 -> [w563 _ _ _ _ _ _ _ _]
              tunnel: w555 -> [w562 _ _ _ _ _ _ _ _]
              tunnel: w554 -> [w561 _ _ _ _ _ _ _ _]
              tunnel: w553 -> [_ w566 _ _ _ _ _ _ _]
              tunnel: w552 -> [_ w565 _ _ _ _ _ _ _]
              tunnel: w551 -> [_ w564 _ _ _ _ _ _ _]
              tunnel: w550 -> [_ _ w569 _ _ _ _ _ _]
              tunnel: w549 -> [_ _ w568 _ _ _ _ _ _]
              tunnel: w548 -> [_ _ w567 _ _ _ _ _ _]
              frame 0, Default {
              }
              frame 1 {
              }
              frame 2 {
              }
              frame 3 {
              }
              frame 4 {
              }
              frame 5 {
              }
              frame 6 {
              }
              frame 7 {
              }
              frame 8 {
              }
            }
          }
        }
        n80 = case shown="8" w113 {
          tunnel: w116 -> [w143 w169 w195 w221 w247 w273 w299 w325 w351]
          tunnel: w115 -> [w142 w168 w194 w220 w246 w272 w298 w324 w350]
          tunnel: w114 -> [w141 w167 w193 w219 w245 w271 w297 w323 w349]
          tunnel: w113 -> [w119 w145 w171 w197 w223 w249 w275 w301 w327]
          frame 0, Default {
            # "you need to unpack each output seperately"
            n81 = call <vilib>:"New Session.vi"("Path to Python Module (.py File)"=path "C:/Users/User/Documents/LabVIEW Data/2015 Projects/LabVIEW Python script/Process Variables/RandomConcGenerator.py") -> ("error out"=w120:errorcluster, "Session ID out"=w137:T4)  [unwired: 9 in]
            n82 = call <vilib>:"Pack.vi"("Argument"=w119, "error in (no error)"=w120, "Session ID"=w137) -> ("error out"=w121:errorcluster, "Python Object References Out"=w122:T5, "Session ID out"=w123:T4)  [unwired: 6 in]
            n83 = call <vilib>:"Pack.vi"("Argument"=2, "error in (no error)"=w121, "Python Object References In"=w122, "Session ID"=w123) -> ("error out"=w125:errorcluster, "Python Object References Out"=w139:T5, "Session ID out"=w140:T4)  [unwired: 5 in]
            n84 = call <vilib>:"Call.vi"("Function or Method Name"="Random", "error in (no error)"=w125, "Python Object References In"=w139, "Session ID"=w140) -> ("error out"=w130:errorcluster, "Python Object References Out"=w131:T5, "Session ID out"=w132:T4)  [unwired: 5 in]
            n85 = call-poly <vilib>:"Unpack.vi"("error in (no error)"=w130, "Python Object References In"=w131, "Session ID"=w132) -> ("error out"=w129:errorcluster, "Value"=→"C BAcid 0":dbl, "Python Object References Out"=w134:T5, "Session ID out"=w136:T4)  [unwired: 5 in]
            n86 = call-poly <vilib>:"Unpack.vi"("error in (no error)"=w129, "Python Object References In"=w134, "Session ID"=w136) -> ("error out"=w128:errorcluster, "Value"=→"C EB 0":dbl, "Session ID out"=w135:T4)  [unwired: 5 in, 1 out]
            n87 = call <vilib>:"Close Session.vi"("error in (no error)"=w128, "Session ID"=w135) -> ()  [unwired: 9 in, 1 out]
            "Flow 0" <- w142
            "Conc 0" <- w141
            "Temp 0" <- w143
            "Boolean 0" <- TRUE
          }
          frame 1 {
            # "you need to unpack each output seperately"
            n88 = call <vilib>:"New Session.vi"("Path to Python Module (.py File)"=path "C:/Users/User/Documents/LabVIEW Data/2015 Projects/LabVIEW Python script/Process Variables/RandomConcGenerator.py") -> ("error out"=w146:errorcluster, "Session ID out"=w163:T4)  [unwired: 9 in]
            n89 = call <vilib>:"Pack.vi"("Argument"=w145, "error in (no error)"=w146, "Session ID"=w163) -> ("error out"=w147:errorcluster, "Python Object References Out"=w148:T5, "Session ID out"=w149:T4)  [unwired: 6 in]
            n90 = call <vilib>:"Pack.vi"("Argument"=2, "error in (no error)"=w147, "Python Object References In"=w148, "Session ID"=w149) -> ("error out"=w151:errorcluster, "Python Object References Out"=w165:T5, "Session ID out"=w166:T4)  [unwired: 5 in]
            n91 = call <vilib>:"Call.vi"("Function or Method Name"="Random", "error in (no error)"=w151, "Python Object References In"=w165, "Session ID"=w166) -> ("error out"=w156:errorcluster, "Python Object References Out"=w157:T5, "Session ID out"=w158:T4)  [unwired: 5 in]
            n92 = call-poly <vilib>:"Unpack.vi"("error in (no error)"=w156, "Python Object References In"=w157, "Session ID"=w158) -> ("error out"=w155:errorcluster, "Value"=→"C BAcid 1":dbl, "Python Object References Out"=w160:T5, "Session ID out"=w162:T4)  [unwired: 5 in]
            n93 = call-poly <vilib>:"Unpack.vi"("error in (no error)"=w155, "Python Object References In"=w160, "Session ID"=w162) -> ("error out"=w154:errorcluster, "Value"=→"C EB 1":dbl, "Session ID out"=w161:T4)  [unwired: 5 in, 1 out]
            n94 = call <vilib>:"Close Session.vi"("error in (no error)"=w154, "Session ID"=w161) -> ()  [unwired: 9 in, 1 out]
            "Flow 1" <- w168
            "Conc 1" <- w167
            "Temp 1" <- w169
            "Boolean 1" <- TRUE
          }
          frame 2 {
            # "you need to unpack each output seperately"
            n95 = call <vilib>:"New Session.vi"("Path to Python Module (.py File)"=path "C:/Users/User/Documents/LabVIEW Data/2015 Projects/LabVIEW Python script/Process Variables/RandomConcGenerator.py") -> ("error out"=w172:errorcluster, "Session ID out"=w189:T4)  [unwired: 9 in]
            n96 = call <vilib>:"Pack.vi"("Argument"=w171, "error in (no error)"=w172, "Session ID"=w189) -> ("error out"=w173:errorcluster, "Python Object References Out"=w174:T5, "Session ID out"=w175:T4)  [unwired: 6 in]
            n97 = call <vilib>:"Pack.vi"("Argument"=2, "error in (no error)"=w173, "Python Object References In"=w174, "Session ID"=w175) -> ("error out"=w177:errorcluster, "Python Object References Out"=w191:T5, "Session ID out"=w192:T4)  [unwired: 5 in]
            n98 = call <vilib>:"Call.vi"("Function or Method Name"="Random", "error in (no error)"=w177, "Python Object References In"=w191, "Session ID"=w192) -> ("error out"=w182:errorcluster, "Python Object References Out"=w183:T5, "Session ID out"=w184:T4)  [unwired: 5 in]
            n99 = call-poly <vilib>:"Unpack.vi"("error in (no error)"=w182, "Python Object References In"=w183, "Session ID"=w184) -> ("error out"=w181:errorcluster, "Value"=→"C BAcid 2":dbl, "Python Object References Out"=w186:T5, "Session ID out"=w188:T4)  [unwired: 5 in]
            n100 = call-poly <vilib>:"Unpack.vi"("error in (no error)"=w181, "Python Object References In"=w186, "Session ID"=w188) -> ("error out"=w180:errorcluster, "Value"=→"C EB 2":dbl, "Session ID out"=w187:T4)  [unwired: 5 in, 1 out]
            n101 = call <vilib>:"Close Session.vi"("error in (no error)"=w180, "Session ID"=w187) -> ()  [unwired: 9 in, 1 out]
            "Flow 2" <- w194
            "Conc 2" <- w193
            "Temp 2" <- w195
            "Boolean 2" <- TRUE
          }
          frame 3 {
            # "you need to unpack each output seperately"
            n102 = call <vilib>:"New Session.vi"("Path to Python Module (.py File)"=path "C:/Users/User/Documents/LabVIEW Data/2015 Projects/LabVIEW Python script/Process Variables/RandomConcGenerator.py") -> ("error out"=w198:errorcluster, "Session ID out"=w215:T4)  [unwired: 9 in]
            n103 = call <vilib>:"Pack.vi"("Argument"=w197, "error in (no error)"=w198, "Session ID"=w215) -> ("error out"=w199:errorcluster, "Python Object References Out"=w200:T5, "Session ID out"=w201:T4)  [unwired: 6 in]
            n104 = call <vilib>:"Pack.vi"("Argument"=2, "error in (no error)"=w199, "Python Object References In"=w200, "Session ID"=w201) -> ("error out"=w203:errorcluster, "Python Object References Out"=w217:T5, "Session ID out"=w218:T4)  [unwired: 5 in]
            n105 = call <vilib>:"Call.vi"("Function or Method Name"="Random", "error in (no error)"=w203, "Python Object References In"=w217, "Session ID"=w218) -> ("error out"=w208:errorcluster, "Python Object References Out"=w209:T5, "Session ID out"=w210:T4)  [unwired: 5 in]
            n106 = call-poly <vilib>:"Unpack.vi"("error in (no error)"=w208, "Python Object References In"=w209, "Session ID"=w210) -> ("error out"=w207:errorcluster, "Value"=→"C BAcid 3":dbl, "Python Object References Out"=w212:T5, "Session ID out"=w214:T4)  [unwired: 5 in]
            n107 = call-poly <vilib>:"Unpack.vi"("error in (no error)"=w207, "Python Object References In"=w212, "Session ID"=w214) -> ("error out"=w206:errorcluster, "Value"=→"C EB 3":dbl, "Session ID out"=w213:T4)  [unwired: 5 in, 1 out]
            n108 = call <vilib>:"Close Session.vi"("error in (no error)"=w206, "Session ID"=w213) -> ()  [unwired: 9 in, 1 out]
            "Flow 3" <- w220
            "Conc 3" <- w219
            "Temp 3" <- w221
            "Boolean 3" <- TRUE
          }
          frame 4 {
            # "you need to unpack each output seperately"
            n109 = call <vilib>:"New Session.vi"("Path to Python Module (.py File)"=path "C:/Users/User/Documents/LabVIEW Data/2015 Projects/LabVIEW Python script/Process Variables/RandomConcGenerator.py") -> ("error out"=w224:errorcluster, "Session ID out"=w241:T4)  [unwired: 9 in]
            n110 = call <vilib>:"Pack.vi"("Argument"=w223, "error in (no error)"=w224, "Session ID"=w241) -> ("error out"=w225:errorcluster, "Python Object References Out"=w226:T5, "Session ID out"=w227:T4)  [unwired: 6 in]
            n111 = call <vilib>:"Pack.vi"("Argument"=2, "error in (no error)"=w225, "Python Object References In"=w226, "Session ID"=w227) -> ("error out"=w229:errorcluster, "Python Object References Out"=w243:T5, "Session ID out"=w244:T4)  [unwired: 5 in]
            n112 = call <vilib>:"Call.vi"("Function or Method Name"="Random", "error in (no error)"=w229, "Python Object References In"=w243, "Session ID"=w244) -> ("error out"=w234:errorcluster, "Python Object References Out"=w235:T5, "Session ID out"=w236:T4)  [unwired: 5 in]
            n113 = call-poly <vilib>:"Unpack.vi"("error in (no error)"=w234, "Python Object References In"=w235, "Session ID"=w236) -> ("error out"=w233:errorcluster, "Value"=→"C BAcid 4":dbl, "Python Object References Out"=w238:T5, "Session ID out"=w240:T4)  [unwired: 5 in]
            n114 = call-poly <vilib>:"Unpack.vi"("error in (no error)"=w233, "Python Object References In"=w238, "Session ID"=w240) -> ("error out"=w232:errorcluster, "Value"=→"C EB 4":dbl, "Session ID out"=w239:T4)  [unwired: 5 in, 1 out]
            n115 = call <vilib>:"Close Session.vi"("error in (no error)"=w232, "Session ID"=w239) -> ()  [unwired: 9 in, 1 out]
            "Flow 4" <- w246
            "Conc 4" <- w245
            "Temp 4" <- w247
            "Boolean 4" <- TRUE
          }
          frame 5 {
            # "you need to unpack each output seperately"
            n116 = call <vilib>:"New Session.vi"("Path to Python Module (.py File)"=path "C:/Users/User/Documents/LabVIEW Data/2015 Projects/LabVIEW Python script/Process Variables/RandomConcGenerator.py") -> ("error out"=w250:errorcluster, "Session ID out"=w267:T4)  [unwired: 9 in]
            n117 = call <vilib>:"Pack.vi"("Argument"=w249, "error in (no error)"=w250, "Session ID"=w267) -> ("error out"=w251:errorcluster, "Python Object References Out"=w252:T5, "Session ID out"=w253:T4)  [unwired: 6 in]
            n118 = call <vilib>:"Pack.vi"("Argument"=2, "error in (no error)"=w251, "Python Object References In"=w252, "Session ID"=w253) -> ("error out"=w255:errorcluster, "Python Object References Out"=w269:T5, "Session ID out"=w270:T4)  [unwired: 5 in]
            n119 = call <vilib>:"Call.vi"("Function or Method Name"="Random", "error in (no error)"=w255, "Python Object References In"=w269, "Session ID"=w270) -> ("error out"=w260:errorcluster, "Python Object References Out"=w261:T5, "Session ID out"=w262:T4)  [unwired: 5 in]
            n120 = call-poly <vilib>:"Unpack.vi"("error in (no error)"=w260, "Python Object References In"=w261, "Session ID"=w262) -> ("error out"=w259:errorcluster, "Value"=→"C BAcid 5":dbl, "Python Object References Out"=w264:T5, "Session ID out"=w266:T4)  [unwired: 5 in]
            n121 = call-poly <vilib>:"Unpack.vi"("error in (no error)"=w259, "Python Object References In"=w264, "Session ID"=w266) -> ("error out"=w258:errorcluster, "Value"=→"C EB 5":dbl, "Session ID out"=w265:T4)  [unwired: 5 in, 1 out]
            n122 = call <vilib>:"Close Session.vi"("error in (no error)"=w258, "Session ID"=w265) -> ()  [unwired: 9 in, 1 out]
            "Flow 5" <- w272
            "Conc 5" <- w271
            "Temp 5" <- w273
            "Boolean 5" <- TRUE
          }
          frame 6 {
            # "you need to unpack each output seperately"
            n123 = call <vilib>:"New Session.vi"("Path to Python Module (.py File)"=path "C:/Users/User/Documents/LabVIEW Data/2015 Projects/LabVIEW Python script/Process Variables/RandomConcGenerator.py") -> ("error out"=w276:errorcluster, "Session ID out"=w293:T4)  [unwired: 9 in]
            n124 = call <vilib>:"Pack.vi"("Argument"=w275, "error in (no error)"=w276, "Session ID"=w293) -> ("error out"=w277:errorcluster, "Python Object References Out"=w278:T5, "Session ID out"=w279:T4)  [unwired: 6 in]
            n125 = call <vilib>:"Pack.vi"("Argument"=2, "error in (no error)"=w277, "Python Object References In"=w278, "Session ID"=w279) -> ("error out"=w281:errorcluster, "Python Object References Out"=w295:T5, "Session ID out"=w296:T4)  [unwired: 5 in]
            n126 = call <vilib>:"Call.vi"("Function or Method Name"="Random", "error in (no error)"=w281, "Python Object References In"=w295, "Session ID"=w296) -> ("error out"=w286:errorcluster, "Python Object References Out"=w287:T5, "Session ID out"=w288:T4)  [unwired: 5 in]
            n127 = call-poly <vilib>:"Unpack.vi"("error in (no error)"=w286, "Python Object References In"=w287, "Session ID"=w288) -> ("error out"=w285:errorcluster, "Value"=→"C BAcid 6":dbl, "Python Object References Out"=w290:T5, "Session ID out"=w292:T4)  [unwired: 5 in]
            n128 = call-poly <vilib>:"Unpack.vi"("error in (no error)"=w285, "Python Object References In"=w290, "Session ID"=w292) -> ("error out"=w284:errorcluster, "Value"=→"C EB 6":dbl, "Session ID out"=w291:T4)  [unwired: 5 in, 1 out]
            n129 = call <vilib>:"Close Session.vi"("error in (no error)"=w284, "Session ID"=w291) -> ()  [unwired: 9 in, 1 out]
            "Flow 6" <- w298
            "Conc 6" <- w297
            "Temp 6" <- w299
            "Boolean 6" <- TRUE
          }
          frame 7 {
            # "you need to unpack each output seperately"
            n130 = call <vilib>:"New Session.vi"("Path to Python Module (.py File)"=path "C:/Users/User/Documents/LabVIEW Data/2015 Projects/LabVIEW Python script/Process Variables/RandomConcGenerator.py") -> ("error out"=w302:errorcluster, "Session ID out"=w319:T4)  [unwired: 9 in]
            n131 = call <vilib>:"Pack.vi"("Argument"=w301, "error in (no error)"=w302, "Session ID"=w319) -> ("error out"=w303:errorcluster, "Python Object References Out"=w304:T5, "Session ID out"=w305:T4)  [unwired: 6 in]
            n132 = call <vilib>:"Pack.vi"("Argument"=2, "error in (no error)"=w303, "Python Object References In"=w304, "Session ID"=w305) -> ("error out"=w307:errorcluster, "Python Object References Out"=w321:T5, "Session ID out"=w322:T4)  [unwired: 5 in]
            n133 = call <vilib>:"Call.vi"("Function or Method Name"="Random", "error in (no error)"=w307, "Python Object References In"=w321, "Session ID"=w322) -> ("error out"=w312:errorcluster, "Python Object References Out"=w313:T5, "Session ID out"=w314:T4)  [unwired: 5 in]
            n134 = call-poly <vilib>:"Unpack.vi"("error in (no error)"=w312, "Python Object References In"=w313, "Session ID"=w314) -> ("error out"=w311:errorcluster, "Value"=→"C BAcid 7":dbl, "Python Object References Out"=w316:T5, "Session ID out"=w318:T4)  [unwired: 5 in]
            n135 = call-poly <vilib>:"Unpack.vi"("error in (no error)"=w311, "Python Object References In"=w316, "Session ID"=w318) -> ("error out"=w310:errorcluster, "Value"=→"C EB 7":dbl, "Session ID out"=w317:T4)  [unwired: 5 in, 1 out]
            n136 = call <vilib>:"Close Session.vi"("error in (no error)"=w310, "Session ID"=w317) -> ()  [unwired: 9 in, 1 out]
            "Flow 7" <- w324
            "Conc 7" <- w323
            "Temp 7" <- w325
            "Boolean 7" <- TRUE
          }
          frame 8 {
            # "you need to unpack each output seperately"
            n137 = call <vilib>:"New Session.vi"("Path to Python Module (.py File)"=path "C:/Users/User/Documents/LabVIEW Data/2015 Projects/LabVIEW Python script/Process Variables/RandomConcGenerator.py") -> ("error out"=w328:errorcluster, "Session ID out"=w345:T4)  [unwired: 9 in]
            n138 = call <vilib>:"Pack.vi"("Argument"=w327, "error in (no error)"=w328, "Session ID"=w345) -> ("error out"=w329:errorcluster, "Python Object References Out"=w330:T5, "Session ID out"=w331:T4)  [unwired: 6 in]
            n139 = call <vilib>:"Pack.vi"("Argument"=2, "error in (no error)"=w329, "Python Object References In"=w330, "Session ID"=w331) -> ("error out"=w333:errorcluster, "Python Object References Out"=w347:T5, "Session ID out"=w348:T4)  [unwired: 5 in]
            n140 = call <vilib>:"Call.vi"("Function or Method Name"="Random", "error in (no error)"=w333, "Python Object References In"=w347, "Session ID"=w348) -> ("error out"=w338:errorcluster, "Python Object References Out"=w339:T5, "Session ID out"=w340:T4)  [unwired: 5 in]
            n141 = call-poly <vilib>:"Unpack.vi"("error in (no error)"=w338, "Python Object References In"=w339, "Session ID"=w340) -> ("error out"=w337:errorcluster, "Value"=→"C BAcid 8":dbl, "Python Object References Out"=w342:T5, "Session ID out"=w344:T4)  [unwired: 5 in]
            n142 = call-poly <vilib>:"Unpack.vi"("error in (no error)"=w337, "Python Object References In"=w342, "Session ID"=w344) -> ("error out"=w336:errorcluster, "Value"=→"C EB 8":dbl, "Session ID out"=w343:T4)  [unwired: 5 in, 1 out]
            n143 = call <vilib>:"Close Session.vi"("error in (no error)"=w336, "Session ID"=w343) -> ()  [unwired: 9 in, 1 out]
            "Flow 8" <- w350
            "Conc 8" <- w349
            "Temp 8" <- w351
            "Boolean 8" <- TRUE
          }
        }
      }
      frame True {
        w588 = 0
      }
    }
    n144 = timed-loop {
      tunnel: w103 -> [w783]
      tunnel: w102 -> [w782]
      tunnel: [w731] -> w101
      tunnel: [w730] -> w100
      timing: w99 -> [_]
      timing-out: [_] -> w98
      tunnel: w97 -> [w717]
      tunnel: w96 -> [w721]
      tunnel: w95 -> [w720]
      tunnel: [w716] -> w94
      tunnel: [w715] -> w93
      tunnel: [w695] -> w92
      tunnel: w83 -> [w712]
      tunnel: w82 -> [w711]
      tunnel: w81 -> [w642]
      tunnel: w91 -> [w700]
      tunnel: w90 -> [w699]
      tunnel: w89 -> [w698]
      tunnel: w88 -> [w697]
      shift-right: [w649] -> _
      shift-left: _ -> [w689]
      tunnel: [w692] -> w87
      tunnel: [w691] -> w86
      tunnel: ["Stop everything"] -> w84
      tunnel: "Automated Experiments or Direct Control" -> [w651]
      i -> [w674]
      stop <- w682 stop-if-true
      w696 = 9.0 ("Safety Shut Down Pressure (barg)")
      w713 = 180
      # "in case out of range changes conc to within possible range"
      # "1st 4 flowrates\n5,6 temperatures\n7 pressure (1)\n8 gas (1)"
      # "temperature or syringe or pressure"
      # "We are graphing in barg"
      # "temperature or syringe"
      # "Empty Syringe has level of 50"
      n145 = node-c288() -> ()  [unwired: 1 in, 1 out]
      n146 = case shown="True" "Change New Set Points" {
        frame False {
        }
        frame True {
          w1163 = 20
          w1157 = ","
          n147 = Divide(x="Set Point 1", y=w1163) -> (x/y=w1140:dbl)
          n148 = Divide(x="Set Point 2", y=w1163) -> (x/y=w1142:dbl)
          n149 = Divide(x="Set Point 3", y=w1163) -> (x/y=w1144:dbl)
          n150 = Divide(x="Set Point 4", y=w1163) -> (x/y=w1146:dbl)
          n151 = Multiply(x=w1140, y=100) -> (x*y=w1152:dbl)
          n152 = Multiply(x=w1142, y=100) -> (x*y=w1153:dbl)
          n153 = Multiply(x=w1144, y=100) -> (x*y=w1154:dbl)
          n154 = Multiply(x=w1146, y=100) -> (x*y=w1155:dbl)
          n155 = Format Into String(w1153) -> (resulting string=w1160:string)  [unwired: 3 in, 1 out]
          n156 = Format Into String(w1152) -> (resulting string=w1159:string)  [unwired: 3 in, 1 out]
          n157 = Format Into String(w1154) -> (resulting string=w1161:string)  [unwired: 3 in, 1 out]
          n158 = Format Into String(w1155) -> (resulting string=w1162:string)  [unwired: 3 in, 1 out]
          n159 = Concatenate Strings("?BSI_SetFlowSetPoints ", w1159, w1157, w1160, w1157, w1161, w1157, w1162, w1157, "*,*,*,*,*,*,*,*,*,*,*,*,*,*,*,*,*,*,*,*,*,*,*,*,*,*") -> (w1139:string)
          n160 = stacked-sequence {
            seq-local: [w1164 _ _] -> [_ _ w1197]
            tunnel: w1139 -> [w1164 _ _]
            frame #0 {
              # "Write Text to Clipboard"
              n161 = String Length(string=w1164) -> (length=w1173:i32)
              n162 = Increment(x=w1173) -> (x+1=w1169:i32)
              n163 = dll-call lib="kernel32" fn="GlobalAlloc"("Flags"=i16 0 ("Format"), "Size"=w1169) -> (w1168:i32)  [unwired: 5 in, 2 out]
              n164 = dll-call lib="kernel32" fn="GlobalLock"("hGlobalMemory"=w1168) -> (w1171:i32)  [unwired: 4 in, 2 out]
              n165 = dll-call lib="kernel32" fn="lstrcpy"("Flags"=w1171, "String"=w1164) -> (w1170:i32)  [unwired: 5 in, 2 out]
              n166 = stacked-sequence {
                tunnel: w1170 -> [_]
                tunnel: w1168 -> [w1192]
                tunnel: [w1191] -> w1167
                frame #0 {
                  n167 = dll-call lib="kernel32" fn="LocalUnlock"("hGlobalMemory"=w1192) -> (w1191:i32)  [unwired: 4 in, 2 out]
                }
              }
              "Error Out 4" <- w1167
              n168 = case shown="0" w1167 {
                selector: w1167 -> [_ w1188]
                tunnel: w1168 -> [w1174 _]
                tunnel: [w1175 w1187] -> w1166
                frame 0 {
                  n169 = dll-call lib="user32" fn="OpenClipboard"("owner"=i16 0) -> (w1176:i32)  [unwired: 4 in, 2 out]
                  n170 = case shown="1, Default" w1176 {
                    selector: w1176 -> [w1180 _]
                    tunnel: [w1178 w1183] -> w1175
                    tunnel: w1174 -> [_ w1182]
                    frame 0 {
                      n171 = Equal To 0?(x=w1180) -> (x = 0?=w1181:bool)
                      n172 = Bundle(w1181, w1180, "source"="Error opening clipboard") -> (w1178:cluster{bool, i32, "source":string})  [unwired: 1 in]
                    }
                    frame 1, Default {
                      n173 = stacked-sequence {
                        tunnel: [_ _ _ cluster{bool, i32, "source":string} {FALSE, 0, "source"=""} ("Output Element")] -> w1183
                        tunnel: w1182 -> [_ w1184 _ _]
                        frame #0 {
                          n174 = dll-call lib="user32" fn="EmptyClipboard"() -> ()  [unwired: 4 in, 2 out]
                        }
                        frame #1 {
                          n175 = dll-call lib="user32" fn="SetClipboardData"("Format"=1, "Data"=w1184) -> ()  [unwired: 6 in, 2 out]
                        }
                        frame #2 {
                          n176 = dll-call lib="user32" fn="CloseClipboard"() -> ()  [unwired: 4 in, 2 out]
                        }
                        frame #3 {
                        }
                      }
                    }
                  }
                }
                frame 1, Default {
                  n177 = Not Equal To 0?(x=w1188) -> (x != 0?=w1189:bool)
                  n178 = Bundle(w1189, w1188, "source"="Error copying text to clipboard") -> (w1187:cluster{bool, i32, "source":string})  [unwired: 1 in]
                }
              }
              "Write error out 4" <- w1166
              n179 = local write "Write Set Point Status"("Running" ("Status")) -> ()
            }
            frame #1 {
              # "Wait 500 milliseconds"
              n180 = Wait (ms)(milliseconds to wait=u32 500) -> ()  [unwired: 1 out]
            }
            frame #2 {
              # "Read Text From Clipboard"
              n181 = dll-call lib="user32" fn="OpenClipboard"("owner"=i16 0) -> (w1199:i32)  [unwired: 4 in, 2 out]
              n182 = case shown="1, Default" w1199 {
                selector: w1199 -> [w1205 _]
                tunnel: ["" w1210] -> w1194
                tunnel: [w1203 cluster{bool, i32, "source":string} {FALSE, 0, "source"=""} ("Output Element")] -> w1198
                frame 0 {
                  n183 = Equal To 0?(x=w1205) -> (x = 0?=w1206:bool)
                  n184 = Bundle(w1206, w1205, "source"="No text in clipboard available!") -> (w1203:cluster{bool, i32, "source":string})  [unwired: 1 in]
                }
                frame 1, Default {
                  n185 = dll-call lib="user32" fn="GetClipboardData"("uFormat"=1 ("hGlobalMemory")) -> (w1211:i32)  [unwired: 4 in, 2 out]
                  n186 = dll-call lib="kernel32" fn="GlobalLock"("hGlobalMemory"=w1211) -> (w1210:string, "hGlobalMemory"=w1208:i32)  [unwired: 3 in, 2 out]
                  n187 = stacked-sequence {
                    tunnel: w1208 -> [w1213 _]
                    frame #0 {
                      n188 = dll-call lib="kernel32" fn="LocalUnlock"("hGlobalMemory"=w1213) -> ()  [unwired: 5 in, 2 out]
                    }
                    frame #1 {
                      n189 = dll-call lib="user32" fn="CloseClipboard"() -> ()  [unwired: 4 in, 2 out]
                    }
                  }
                }
              }
              "Text Read From Clipboard 4" <- w1194
              "Read error out 4" <- w1198
              n190 = Equal?(x=w1197, y=w1194) -> (x = y?=w1196:bool)
              n191 = case shown="True" w1196 {
                tunnel: ["Response OK" "Failed: No Response from Lab Interface"] -> w1195
                frame False {
                }
                frame True {
                }
              }
              "Write Set Point Status" <- w1195
            }
          }
        }
      }
      n192 = Or(x="Read Set Points", y="Change New Set Points") -> (x .or. y?=w687:bool)
      n193 = Or(x="Test Gas Communication", y=w687) -> (x .or. y?=w684:bool)
      n194 = case shown="True" "Test Gas Communication" {
        frame False {
        }
        frame True {
          w1088 = "?BSI_Test"  # ?BSI_Test
          n195 = stacked-sequence {
            seq-local: [w1089 _ _] -> [_ _ w1122]
            tunnel: w1088 -> [w1089 _ _]
            frame #0 {
              # "Write Text to Clipboard"
              n196 = String Length(string=w1089) -> (length=w1098:i32)
              n197 = Increment(x=w1098) -> (x+1=w1094:i32)
              n198 = dll-call lib="kernel32" fn="GlobalAlloc"("Flags"=i16 0 ("Format"), "Size"=w1094) -> (w1093:i32)  [unwired: 5 in, 2 out]
              n199 = dll-call lib="kernel32" fn="GlobalLock"("hGlobalMemory"=w1093) -> (w1096:i32)  [unwired: 4 in, 2 out]
              n200 = dll-call lib="kernel32" fn="lstrcpy"("Flags"=w1096, "String"=w1089) -> (w1095:i32)  [unwired: 5 in, 2 out]
              n201 = stacked-sequence {
                tunnel: w1095 -> [_]
                tunnel: w1093 -> [w1117]
                tunnel: [w1116] -> w1092
                frame #0 {
                  n202 = dll-call lib="kernel32" fn="LocalUnlock"("hGlobalMemory"=w1117) -> (w1116:i32)  [unwired: 4 in, 2 out]
                }
              }
              "Error Out" <- w1092
              n203 = case shown="1, Default" w1092 {
                selector: w1092 -> [_ w1113]
                tunnel: w1093 -> [w1099 _]
                tunnel: [w1100 w1112] -> w1091
                frame 0 {
                  n204 = dll-call lib="user32" fn="OpenClipboard"("owner"=i16 0) -> (w1101:i32)  [unwired: 4 in, 2 out]
                  n205 = case shown="0" w1101 {
                    selector: w1101 -> [w1105 _]
                    tunnel: [w1103 w1108] -> w1100
                    tunnel: w1099 -> [_ w1107]
                    frame 0 {
                      n206 = Equal To 0?(x=w1105) -> (x = 0?=w1106:bool)
                      n207 = Bundle(w1106, w1105, "source"="Error opening clipboard") -> (w1103:cluster{bool, i32, "source":string})  [unwired: 1 in]
                    }
                    frame 1, Default {
                      n208 = stacked-sequence {
                        tunnel: [_ _ _ cluster{bool, i32, "source":string} {FALSE, 0, "source"=""} ("Output Element")] -> w1108
                        tunnel: w1107 -> [_ w1109 _ _]
                        frame #0 {
                          n209 = dll-call lib="user32" fn="EmptyClipboard"() -> ()  [unwired: 4 in, 2 out]
                        }
                        frame #1 {
                          n210 = dll-call lib="user32" fn="SetClipboardData"("Format"=1, "Data"=w1109) -> ()  [unwired: 6 in, 2 out]
                        }
                        frame #2 {
                          n211 = dll-call lib="user32" fn="CloseClipboard"() -> ()  [unwired: 4 in, 2 out]
                        }
                        frame #3 {
                        }
                      }
                    }
                  }
                }
                frame 1, Default {
                  n212 = Not Equal To 0?(x=w1113) -> (x != 0?=w1114:bool)
                  n213 = Bundle(w1114, w1113, "source"="Error copying text to clipboard") -> (w1112:cluster{bool, i32, "source":string})  [unwired: 1 in]
                }
              }
              "Write error out" <- w1091
              n214 = local write "Test Status"("Running" ("Status")) -> ()
            }
            frame #1 {
              # "Wait 500 milliseconds"
              n215 = Wait (ms)(milliseconds to wait=u32 500) -> ()  [unwired: 1 out]
            }
            frame #2 {
              # "Read Text From Clipboard"
              n216 = dll-call lib="user32" fn="OpenClipboard"("owner"=i16 0) -> (w1124:i32)  [unwired: 4 in, 2 out]
              n217 = case shown="1, Default" w1124 {
                selector: w1124 -> [w1130 _]
                tunnel: ["" w1135] -> w1119
                tunnel: [w1128 cluster{bool, i32, "source":string} {FALSE, 0, "source"=""} ("Output Element")] -> w1123
                frame 0 {
                  n218 = Equal To 0?(x=w1130) -> (x = 0?=w1131:bool)
                  n219 = Bundle(w1131, w1130, "source"="No text in clipboard available!") -> (w1128:cluster{bool, i32, "source":string})  [unwired: 1 in]
                }
                frame 1, Default {
                  n220 = dll-call lib="user32" fn="GetClipboardData"("uFormat"=1 ("hGlobalMemory")) -> (w1136:i32)  [unwired: 4 in, 2 out]
                  n221 = dll-call lib="kernel32" fn="GlobalLock"("hGlobalMemory"=w1136) -> (w1135:string, "hGlobalMemory"=w1133:i32)  [unwired: 3 in, 2 out]
                  n222 = stacked-sequence {
                    tunnel: w1133 -> [w1138 _]
                    frame #0 {
                      n223 = dll-call lib="kernel32" fn="LocalUnlock"("hGlobalMemory"=w1138) -> ()  [unwired: 5 in, 2 out]
                    }
                    frame #1 {
                      n224 = dll-call lib="user32" fn="CloseClipboard"() -> ()  [unwired: 4 in, 2 out]
                    }
                  }
                }
              }
              "Text Read From Clipboard" <- w1119
              "Read error out" <- w1123
              n225 = Equal?(x=w1122, y=w1119) -> (x = y?=w1121:bool)
              n226 = case shown="True" w1121 {
                tunnel: ["Response OK" "Failed: No Response from Lab Interface"] -> w1120
                frame False {
                }
                frame True {
                }
              }
              "Test Status" <- w1120
            }
          }
        }
      }
      n227 = case shown="True" "Read Set Points" {
        frame False {
        }
        frame True {
          w962 = "?BSI_ReadFlowSetPoints"  # ?BSI_ReadFlowSetPoints
          n228 = stacked-sequence {
            seq-local: [w963 _ _] -> [_ _ w996]
            tunnel: w962 -> [w963 _ _]
            frame #0 {
              # "Write Text to Clipboard"
              n229 = String Length(string=w963) -> (length=w972:i32)
              n230 = Increment(x=w972) -> (x+1=w968:i32)
              n231 = dll-call lib="kernel32" fn="GlobalAlloc"("Flags"=i16 0 ("Format"), "Size"=w968) -> (w967:i32)  [unwired: 5 in, 2 out]
              n232 = dll-call lib="kernel32" fn="GlobalLock"("hGlobalMemory"=w967) -> (w970:i32)  [unwired: 4 in, 2 out]
              n233 = dll-call lib="kernel32" fn="lstrcpy"("Flags"=w970, "String"=w963) -> (w969:i32)  [unwired: 5 in, 2 out]
              n234 = stacked-sequence {
                tunnel: w969 -> [_]
                tunnel: w967 -> [w991]
                tunnel: [w990] -> w966
                frame #0 {
                  n235 = dll-call lib="kernel32" fn="LocalUnlock"("hGlobalMemory"=w991) -> (w990:i32)  [unwired: 4 in, 2 out]
                }
              }
              "Error Out 3" <- w966
              n236 = case shown="0" w966 {
                selector: w966 -> [_ w987]
                tunnel: w967 -> [w973 _]
                tunnel: [w974 w986] -> w965
                frame 0 {
                  n237 = dll-call lib="user32" fn="OpenClipboard"("owner"=i16 0) -> (w975:i32)  [unwired: 4 in, 2 out]
                  n238 = case shown="1, Default" w975 {
                    selector: w975 -> [w979 _]
                    tunnel: [w977 w982] -> w974
                    tunnel: w973 -> [_ w981]
                    frame 0 {
                      n239 = Equal To 0?(x=w979) -> (x = 0?=w980:bool)
                      n240 = Bundle(w980, w979, "source"="Error opening clipboard") -> (w977:cluster{bool, i32, "source":string})  [unwired: 1 in]
                    }
                    frame 1, Default {
                      n241 = stacked-sequence {
                        tunnel: [_ _ _ cluster{bool, i32, "source":string} {FALSE, 0, "source"=""} ("Output Element")] -> w982
                        tunnel: w981 -> [_ w983 _ _]
                        frame #0 {
                          n242 = dll-call lib="user32" fn="EmptyClipboard"() -> ()  [unwired: 4 in, 2 out]
                        }
                        frame #1 {
                          n243 = dll-call lib="user32" fn="SetClipboardData"("Format"=1, "Data"=w983) -> ()  [unwired: 6 in, 2 out]
                        }
                        frame #2 {
                          n244 = dll-call lib="user32" fn="CloseClipboard"() -> ()  [unwired: 4 in, 2 out]
                        }
                        frame #3 {
                        }
                      }
                    }
                  }
                }
                frame 1, Default {
                  n245 = Not Equal To 0?(x=w987) -> (x != 0?=w988:bool)
                  n246 = Bundle(w988, w987, "source"="Error copying text to clipboard") -> (w986:cluster{bool, i32, "source":string})  [unwired: 1 in]
                }
              }
              "Write error out 3" <- w965
              n247 = local write "Read Set Point Status"("Running" ("Status")) -> ()
            }
            frame #1 {
              # "Wait 500 milliseconds"
              n248 = Wait (ms)(milliseconds to wait=u32 500) -> ()  [unwired: 1 out]
            }
            frame #2 {
              # "Read Text From Clipboard"
              n249 = dll-call lib="user32" fn="OpenClipboard"("owner"=i16 0) -> (w998:i32)  [unwired: 4 in, 2 out]
              n250 = case shown="1, Default" w998 {
                selector: w998 -> [w1004 _]
                tunnel: ["" w1009] -> w993
                tunnel: [w1002 cluster{bool, i32, "source":string} {FALSE, 0, "source"=""} ("Output Element")] -> w997
                frame 0 {
                  n251 = Equal To 0?(x=w1004) -> (x = 0?=w1005:bool)
                  n252 = Bundle(w1005, w1004, "source"="No text in clipboard available!") -> (w1002:cluster{bool, i32, "source":string})  [unwired: 1 in]
                }
                frame 1, Default {
                  n253 = dll-call lib="user32" fn="GetClipboardData"("uFormat"=1 ("hGlobalMemory")) -> (w1010:i32)  [unwired: 4 in, 2 out]
                  n254 = dll-call lib="kernel32" fn="GlobalLock"("hGlobalMemory"=w1010) -> (w1009:string, "hGlobalMemory"=w1007:i32)  [unwired: 3 in, 2 out]
                  n255 = stacked-sequence {
                    tunnel: w1007 -> [w1012 _]
                    frame #0 {
                      n256 = dll-call lib="kernel32" fn="LocalUnlock"("hGlobalMemory"=w1012) -> ()  [unwired: 5 in, 2 out]
                    }
                    frame #1 {
                      n257 = dll-call lib="user32" fn="CloseClipboard"() -> ()  [unwired: 4 in, 2 out]
                    }
                  }
                }
              }
              "Text Read From Clipboard 3" <- w993
              "Read error out 3" <- w997
              n258 = Equal?(x=w996, y=w993) -> (x = y?=w995:bool)
              n259 = case shown="True" w995 {
                tunnel: ["Response OK" "Failed: No Response from Lab Interface"] -> w994
                frame False {
                }
                frame True {
                }
              }
              "Read Set Point Status" <- w994
            }
          }
        }
      }
      n260 = for {
        N: 4 -> [_]
        tunnel: w783 -> [w1312] mode=indexing
        tunnel: [w1310] -> w777 mode=indexing
        tunnel: [w1307] -> w772 mode=indexing
        tunnel: [w1306] -> w771 mode=indexing
        tunnel: [w1305] -> w770 mode=indexing
        tunnel: w782 -> [w1304] mode=indexing
        i -> [w1311]
        n261 = call "NCS_GetFlowRateIs.vi"("error in (no error)"=w1304, "dosingunit"=w1311, "device handle in"=w1312) -> ("error out"=w1308:errorcluster, "flowrate is"=w1310:dbl, "device handle out"=w1309:u32)
        n262 = call "NCS_GetSyringeLevelIs.vi"("error in (no error)"=w1308, "dosingunit"=w1311, "device handle in"=w1309) -> ("error out"=w1305:errorcluster, "syringe level is"=w1307:dbl, "device handle out"=w1306:u32)
      }
      n263 = Index Array(array=w772, index=0) -> (element=w678:dbl)
      "Syringe Level 1" <- w678
      n264 = Index Array(array=w772, index=3) -> (element=w675:dbl)
      "Syringe Level 4" <- w675
      n265 = Index Array(array=w772, index=1) -> (element=w677:dbl)
      "Syringe Level 2" <- w677
      n266 = Index Array(array=w772, index=2) -> (element=w676:dbl)
      "Syringe Level 3" <- w676
      n267 = case shown="True" "Shut down in empty?\nLeft off, right on" {
        tunnel: [FALSE w954] -> w679
        tunnel: w678 -> [_ w953]
        tunnel: w677 -> [_ w952]
        tunnel: w676 -> [_ w951]
        tunnel: w675 -> [_ w950]
        frame False {
        }
        frame True {
          w955 = 50
          n268 = Less Or Equal?(x=w952, y=w955) -> (x <= y?=w961:bool)
          n269 = Less Or Equal?(x=w953, y=w955) -> (x <= y?=w956:bool)
          n270 = Less Or Equal?(x=w951, y=w955) -> (x <= y?=w959:bool)
          n271 = Less Or Equal?(x=w950, y=w955) -> (x <= y?=w957:bool)
          n272 = Or(x=w956, y=w961) -> (x .or. y?=w960:bool)
          n273 = Or(x=w960, y=w959) -> (x .or. y?=w958:bool)
          n274 = Or(x=w958, y=w957) -> (x .or. y?=w954:bool)
        }
      }
      n275 = Index Array(array=w777, index=0) -> (element=w662:dbl)
      "Flowrate 1 High" <- w662
      n276 = Index Array(array=w777, index=3) -> (element=w664:dbl)
      "Flowrate 4 Ethanol" <- w664
      n277 = Index Array(array=w777, index=1) -> (element=w661:dbl)
      "Flowrate 2 Low" <- w661
      n278 = Index Array(array=w777, index=2) -> (element=w665:dbl)
      "Flowrate 3 Acid" <- w665
      n279 = case shown="True" "Clear" {
        tunnel: w689 -> [w1214 _]
        tunnel: [w1214 w1215] -> w688
        frame False {
        }
        frame True {
          n280 = Initialize Array(0, 1) -> (w1215:i32[])
        }
      }
      n281 = call-poly <vilib>:"DAQmx Read.vi"("task/channels in"=w700, "error in"=w699) -> ("task out"=w692:refnum<k21>, "data"=w705:dbl[], "error out"=w691:errorcluster)  [unwired: 11 in]
      n282 = Add(x=w662, y=w661) -> (x+y=w667:dbl)
      n283 = Add(x=w667, y=w665) -> (x+y=w666:dbl)
      n284 = Index Array(array=w705, index=0) -> (element=w703:dbl)
      n285 = Add(x=w666, y=w664) -> (x+y=w663:dbl)
      "Total Flowrate (uL/min)" <- w663
      n286 = Divide(x=w662, y=w663) -> (x/y=w656:dbl)
      n287 = Multiply(x=w703, y=w698) -> (x*y=w704:dbl)
      n288 = Multiply(x="High Conc", y=w656) -> (x*y=w660:dbl)
      n289 = Add(x=w704, y=w697) -> (x+y=w701:dbl)
      n290 = Divide(x=w661, y=w663) -> (x/y=w657:dbl)
      n291 = Multiply(x="High Conc", y=0.9) -> (x*y=w646:dbl)
      n292 = Multiply(x="Low Conc", y=0.9) -> (x*y=w645:dbl)
      n293 = Multiply(x="Low Conc", y=w657) -> (x*y=w659:dbl)
      n294 = Add(x=w660, y=w659) -> (x+y=→"Feed Concentration (M)":dbl)
      n295 = In Range and Coerce(upper limit=w646, x=w642, lower limit=w645) -> (coerced(x)=w639:dbl, In Range?=w641:bool)
      n296 = case shown="False" w641 {
        tunnel: [w786 w788] -> w640
        tunnel: w642 -> [_ w788]
        tunnel: w639 -> [w786 _]
        tunnel: [TRUE FALSE] -> w638
        frame False {
        }
        frame True {
        }
      }
      "Desired Conc Not Possible" <- w638
      n297 = Multiply(x=w701, y=0.0689476) -> (x*y=w650:dbl)
      "Pressure (barg)" <- w650
      n298 = case shown="False" w651 {
        tunnel: [w1284 w1285] -> w768
        tunnel: w711 -> [w1271 _]
        tunnel: w640 -> [w1273 _]
        tunnel: "High Conc" -> [w1270 _]
        tunnel: "Low Conc" -> [w1269 _]
        frame False {
          w1268 = 0.1
          n299 = Subtract(x=w1270, y=w1269) -> (x-y=w1280:dbl)
          n300 = Subtract(x=1, y=w1268) -> (x-y=w1276:dbl)
          n301 = Divide(x=w1273, y=w1276) -> (x/y=w1282:dbl)
          n302 = Multiply(x=0, y=w1271) -> (x*y=w1264:dbl)
          n303 = Subtract(x=w1270, y=w1282) -> (x-y=w1279:dbl)
          n304 = Subtract(x=w1282, y=w1269) -> (x-y=w1281:dbl)
          n305 = Divide(x=w1281, y=w1280) -> (x/y=w1278:dbl)
          n306 = Divide(x=w1279, y=w1280) -> (x/y=w1277:dbl)
          n307 = Multiply(x=w1278, y=w1276) -> (x*y=w1275:dbl)
          n308 = Multiply(x=w1277, y=w1276) -> (x*y=w1274:dbl)
          n309 = Multiply(x=w1271, y=w1274) -> (x*y=w1266:dbl)
          n310 = Multiply(x=w1271, y=w1275) -> (x*y=w1265:dbl)
          n311 = Multiply(x=w1271, y=w1268) -> (x*y=w1267:dbl)
          n312 = Build Array(w1265, w1266, w1267, w1264) -> (w1284:dbl[])
          "Volumetric Fraction Acid" <- w1268
        }
        frame True {
          n313 = Build Array("Set Flowrate 1", "Set Flowrate 2", "Set Flowrate 3", "Set Flowrate 4") -> (w1285:dbl[])
        }
      }
      n314 = Build Array (concatenate)(w688, w650) -> (w649:dbl[])
      "Calculated Pressure" <- w649
      n315 = Greater Or Equal?(x=w650, y=w696) -> (x >= y?=w693:bool)
      n316 = case shown="True" w651 {
        tunnel: [w1219 FALSE] -> w654
        tunnel: w674 -> [w1218 _]
        frame False {
          # "changes set points for each new exp"
          n317 = Equal?(x=w1218, y=0) -> (x = y?=w1219:bool)
        }
        frame True {
          # "at end of each exp"
          # "doesnt automatically change set point"
        }
      }
      n318 = Or(x=w654, y="Update Temperature Set Point") -> (x .or. y?=w723:bool)
      n319 = case shown="True" w723 {
        tunnel: w721 -> [w1223 w1231]
        tunnel: w720 -> [w1222 w1230]
        tunnel: [w1223 w1229] -> w719
        tunnel: [w1222 w1228] -> w718
        tunnel: w717 -> [_ w1227]
        tunnel: w651 -> [_ w1225]
        tunnel: w712 -> [_ w1224]
        frame False {
        }
        frame True {
          n320 = case shown="True" w1225 {
            tunnel: [w1232 "Set Point (oC)"] -> w1226
            tunnel: w1224 -> [w1232 _]
            frame False {
            }
            frame True {
            }
          }
          n321 = call "CN7500_Write Set Point Value.vi"("Target Set Point Value"=w1226, "error in (no error)"=w1230, "Controller Number"=w1227, "VISA In"=w1231) -> ("error out"=w1228:errorcluster, "VISA Out"=w1229:refnum<visa-resource-name>)  [unwired: 6 in]
        }
      }
      n322 = Or(x="Generate Flow", y=w654) -> (x .or. y?=w655:bool)
      n323 = case shown="True" w655 {
        tunnel: w771 -> [w1291 w1296]
        tunnel: w770 -> [w1290 w1295]
        tunnel: [w1290 w1294] -> w669
        tunnel: [w1291 w1293] -> w668
        tunnel: w768 -> [_ w1292]
        frame False {
        }
        frame True {
          n324 = for {
            N: 4 -> [_]
            tunnel: w1296 -> [w1303] mode=indexing
            tunnel: w1295 -> [w1302] mode=indexing
            tunnel: [w1301] -> w1294 mode=indexing
            tunnel: [w1300] -> w1293 mode=indexing
            tunnel: w1292 -> [w1298] mode=indexing
            i -> [w1299]
            n325 = call "NCS_GenerateFlow.vi"("error in (no error)"=w1302, "flowrate"=w1298, "dosingunit"=w1299, "device handle in"=w1303) -> ("error out"=w1301:errorcluster, "device handle out"=w1300:u32)
          }
        }
      }
      n326 = call "CN7500_Read Process Value.vi"("error in (no error)"=w718, "Controller Number"=w717, "VISA In"=w719) -> ("error out"=w716:errorcluster, "Set Point Value"=w707:dbl, "Process Value"=w708:dbl, "VISA Out"=w715:refnum<visa-resource-name>)  [unwired: 5 in]
      "Temp Set Point (oC)" <- w707
      "Actual Temp (oC)" <- w708
      n327 = Merge Signals(w708, w707) -> (→"Temperature":dynamicdata)
      n328 = Greater Or Equal?(x=w708, y=w713) -> (x >= y?=w710:bool)
      n329 = Index Array(array=w669, index=0) -> (element=w758:errorcluster)
      n330 = Index Array(array=w668, index=0) -> (element=w759:u32)
      n331 = Index Array(array=w669, index=3) -> (element=w748:errorcluster)
      n332 = Index Array(array=w669, index=2) -> (element=w750:errorcluster)
      n333 = Index Array(array=w669, index=1) -> (element=w752:errorcluster)
      n334 = Index Array(array=w668, index=3) -> (element=w749:u32)
      n335 = Index Array(array=w668, index=2) -> (element=w751:u32)
      n336 = Index Array(array=w668, index=1) -> (element=w753:u32)
      n337 = case shown="False" "Stop Dose 2" {
        tunnel: w753 -> [w1251 w1256]
        tunnel: w752 -> [w1250 w1255]
        tunnel: [w1251 w1254] -> w745
        tunnel: [w1250 w1253] -> w744
        frame False {
        }
        frame True {
          n338 = call "NCS_Stop.vi"("error in (no error)"=w1255, "dosingunit"=1, "device handle in"=w1256) -> ("error out"=w1253:errorcluster, "device handle out"=w1254:u32)
        }
      }
      n339 = case shown="False" "Stop Dose 1" {
        tunnel: w759 -> [w1258 w1263]
        tunnel: w758 -> [w1257 w1262]
        tunnel: [w1258 w1261] -> w747
        tunnel: [w1257 w1260] -> w746
        frame False {
        }
        frame True {
          n340 = call "NCS_Stop.vi"("error in (no error)"=w1262, "dosingunit"=0, "device handle in"=w1263) -> ("error out"=w1260:errorcluster, "device handle out"=w1261:u32)
        }
      }
      n341 = case shown="False" "Stop Dose 3" {
        tunnel: w751 -> [w1244 w1249]
        tunnel: w750 -> [w1243 w1248]
        tunnel: [w1244 w1247] -> w743
        tunnel: [w1243 w1246] -> w742
        frame False {
        }
        frame True {
          n342 = call "NCS_Stop.vi"("error in (no error)"=w1248, "dosingunit"=2, "device handle in"=w1249) -> ("error out"=w1246:errorcluster, "device handle out"=w1247:u32)
        }
      }
      n343 = case shown="False" "Stop Dose 4" {
        tunnel: w749 -> [w1237 w1242]
        tunnel: w748 -> [w1236 w1241]
        tunnel: [w1237 w1240] -> w741
        tunnel: [w1236 w1239] -> w740
        frame False {
        }
        frame True {
          n344 = call "NCS_Stop.vi"("error in (no error)"=w1241, "dosingunit"=3, "device handle in"=w1242) -> ("error out"=w1239:errorcluster, "device handle out"=w1240:u32)
        }
      }
      n345 = case shown="False" "Safety or Emergency Syringe Control" {
        tunnel: w747 -> [w796 w837]
        tunnel: w746 -> [w792 w836]
        tunnel: w745 -> [w795 w835]
        tunnel: w744 -> [w791 w834]
        tunnel: w743 -> [w794 w833]
        tunnel: w742 -> [w790 w832]
        tunnel: w741 -> [w793 w831]
        tunnel: w740 -> [w789 w830]
        tunnel: [w796 w807] -> w739
        tunnel: [w795 w806] -> w738
        tunnel: [w794 w805] -> w737
        tunnel: [w793 w804] -> w736
        tunnel: [w791 w803] -> w735
        tunnel: [w790 w802] -> w734
        tunnel: [w789 w801] -> w733
        tunnel: [w792 w797] -> w732
        frame False {
        }
        frame True {
          n346 = case shown="False" "Calibrate 2" {
            tunnel: w835 -> [w936 w941]
            tunnel: w834 -> [w935 w940]
            tunnel: [w936 w939] -> w824
            tunnel: [w935 w938] -> w823
            frame False {
            }
            frame True {
              n347 = call "NCS_Calibrate.vi"("error in (no error)"=w940, "dosingunit"=1, "device handle in"=w941) -> ("error out"=w938:errorcluster, "device handle out"=w939:u32)
            }
          }
          n348 = case shown="False" "Calibrate 3" {
            tunnel: w833 -> [w929 w934]
            tunnel: w832 -> [w928 w933]
            tunnel: [w929 w932] -> w822
            tunnel: [w928 w931] -> w821
            frame False {
            }
            frame True {
              n349 = call "NCS_Calibrate.vi"("error in (no error)"=w933, "dosingunit"=2, "device handle in"=w934) -> ("error out"=w931:errorcluster, "device handle out"=w932:u32)
            }
          }
          n350 = case shown="False" "Calibrate 1" {
            tunnel: w837 -> [w943 w948]
            tunnel: w836 -> [w942 w947]
            tunnel: [w943 w946] -> w826
            tunnel: [w942 w945] -> w825
            frame False {
            }
            frame True {
              n351 = call "NCS_Calibrate.vi"("error in (no error)"=w947, "dosingunit"=0, "device handle in"=w948) -> ("error out"=w945:errorcluster, "device handle out"=w946:u32)
            }
          }
          n352 = case shown="False" "Calibrate 4" {
            tunnel: w831 -> [w922 w927]
            tunnel: w830 -> [w921 w926]
            tunnel: [w922 w925] -> w820
            tunnel: [w921 w924] -> w819
            frame False {
            }
            frame True {
              n353 = call "NCS_Calibrate.vi"("error in (no error)"=w926, "dosingunit"=3, "device handle in"=w927) -> ("error out"=w924:errorcluster, "device handle out"=w925:u32)
            }
          }
          n354 = case shown="False" "Empty 2" {
            tunnel: w824 -> [w902 w906]
            tunnel: w823 -> [w901 w904]
            tunnel: [w902 w905] -> w810
            tunnel: [w901 w903] -> w811
            frame False {
            }
            frame True {
              w908 = 1
              n355 = call "NCS_GetFlowRateMax.vi"("error in (no error)"=w904, "dosingunit"=w908, "device handle in"=w906) -> ("error out"=w909:errorcluster, "flow rate max"=w907:dbl, "device handle out"=w910:u32)
              n356 = call "NCS_EmptySyrige.vi"("error in (no error)"=w909, "flowrate"=w907, "dosingunit"=w908, "device handle in"=w910) -> ("error out"=w903:errorcluster, "device handle out"=w905:u32)
            }
          }
          n357 = case shown="False" "Empty 1" {
            tunnel: w826 -> [w912 w920]
            tunnel: w825 -> [w911 w917]
            tunnel: [w912 w918] -> w808
            tunnel: [w911 w915] -> w809
            frame False {
            }
            frame True {
              w914 = 0
              n358 = call "NCS_GetFlowRateMax.vi"("error in (no error)"=w917, "dosingunit"=w914, "device handle in"=w920) -> ("error out"=w916:errorcluster, "flow rate max"=w913:dbl, "device handle out"=w919:u32)
              n359 = call "NCS_EmptySyrige.vi"("error in (no error)"=w916, "flowrate"=w913, "dosingunit"=w914, "device handle in"=w919) -> ("error out"=w915:errorcluster, "device handle out"=w918:u32)
            }
          }
          n360 = case shown="False" "Empty 3" {
            tunnel: w822 -> [w892 w893]
            tunnel: w821 -> [w891 w894]
            tunnel: [w892 w895] -> w812
            tunnel: [w891 w896] -> w813
            frame False {
            }
            frame True {
              w898 = 2
              n361 = call "NCS_GetFlowRateMax.vi"("error in (no error)"=w894, "dosingunit"=w898, "device handle in"=w893) -> ("error out"=w899:errorcluster, "flow rate max"=w897:dbl, "device handle out"=w900:u32)
              n362 = call "NCS_EmptySyrige.vi"("error in (no error)"=w899, "flowrate"=w897, "dosingunit"=w898, "device handle in"=w900) -> ("error out"=w896:errorcluster, "device handle out"=w895:u32)
            }
          }
          n363 = case shown="False" "Empty 4" {
            tunnel: w820 -> [w882 w883]
            tunnel: w819 -> [w881 w884]
            tunnel: [w882 w886] -> w814
            tunnel: [w881 w885] -> w815
            frame False {
            }
            frame True {
              w888 = 3
              n364 = call "NCS_GetFlowRateMax.vi"("error in (no error)"=w884, "dosingunit"=w888, "device handle in"=w883) -> ("error out"=w889:errorcluster, "flow rate max"=w887:dbl, "device handle out"=w890:u32)
              n365 = call "NCS_EmptySyrige.vi"("error in (no error)"=w889, "flowrate"=w887, "dosingunit"=w888, "device handle in"=w890) -> ("error out"=w885:errorcluster, "device handle out"=w886:u32)
            }
          }
          n366 = case shown="False" "Refill 2" {
            tunnel: w810 -> [w862 w866]
            tunnel: w811 -> [w861 w864]
            tunnel: [w862 w865] -> w806
            tunnel: [w861 w863] -> w803
            frame False {
            }
            frame True {
              w868 = 1
              n367 = call "NCS_GetFlowRateMax.vi"("error in (no error)"=w864, "dosingunit"=w868, "device handle in"=w866) -> ("error out"=w869:errorcluster, "flow rate max"=w867:dbl, "device handle out"=w870:u32)
              n368 = call "NCS_RefillSyrige.vi"("error in (no error)"=w869, "flowrate"=w867, "dosingunit"=w868, "device handle in"=w870) -> ("error out"=w863:errorcluster, "device handle out"=w865:u32)
            }
          }
          n369 = case shown="False" "Refill 1" {
            tunnel: w808 -> [w872 w880]
            tunnel: w809 -> [w871 w877]
            tunnel: [w872 w878] -> w807
            tunnel: [w871 w875] -> w797
            frame False {
            }
            frame True {
              w874 = 0
              n370 = call "NCS_GetFlowRateMax.vi"("error in (no error)"=w877, "dosingunit"=w874, "device handle in"=w880) -> ("error out"=w876:errorcluster, "flow rate max"=w873:dbl, "device handle out"=w879:u32)
              n371 = call "NCS_RefillSyrige.vi"("error in (no error)"=w876, "flowrate"=w873, "dosingunit"=w874, "device handle in"=w879) -> ("error out"=w875:errorcluster, "device handle out"=w878:u32)
            }
          }
          n372 = case shown="False" "Refill 3" {
            tunnel: w812 -> [w852 w853]
            tunnel: w813 -> [w851 w854]
            tunnel: [w852 w855] -> w805
            tunnel: [w851 w856] -> w802
            frame False {
            }
            frame True {
              w858 = 2
              n373 = call "NCS_GetFlowRateMax.vi"("error in (no error)"=w854, "dosingunit"=w858, "device handle in"=w853) -> ("error out"=w859:errorcluster, "flow rate max"=w857:dbl, "device handle out"=w860:u32)
              n374 = call "NCS_RefillSyrige.vi"("error in (no error)"=w859, "flowrate"=w857, "dosingunit"=w858, "device handle in"=w860) -> ("error out"=w856:errorcluster, "device handle out"=w855:u32)
            }
          }
          n375 = case shown="False" "Refill 4" {
            tunnel: w814 -> [w842 w843]
            tunnel: w815 -> [w841 w844]
            tunnel: [w842 w846] -> w804
            tunnel: [w841 w845] -> w801
            frame False {
            }
            frame True {
              w848 = 3
              n376 = call "NCS_GetFlowRateMax.vi"("error in (no error)"=w844, "dosingunit"=w848, "device handle in"=w843) -> ("error out"=w849:errorcluster, "flow rate max"=w847:dbl, "device handle out"=w850:u32)
              n377 = call "NCS_RefillSyrige.vi"("error in (no error)"=w849, "flowrate"=w847, "dosingunit"=w848, "device handle in"=w850) -> ("error out"=w845:errorcluster, "device handle out"=w846:u32)
            }
          }
        }
      }
      n378 = Or(x=w710, y=w679) -> (x .or. y?=w694:bool)
      n379 = Or(x=w694, y=w693) -> (x .or. y?=w695:bool)
      n380 = Multiply(x="Minutes between Exp", y=60) -> (x*y=w671:dbl)
      n381 = Divide(x=w671, y=5) -> (x/y=w672:dbl)
      n382 = Greater Or Equal?(x=w674, y=w672) -> (x >= y?=w725:bool)
      n383 = Or(x=w725, y=w695) -> (x .or. y?=w709:bool)
      n384 = Or(x="Skip Exp", y=w709) -> (x .or. y?=w726:bool)
      n385 = Or(x="Stop everything", y=w726) -> (x .or. y?=w682:bool)
      n386 = Or(x=w682, y=w684) -> (x .or. y?=w683:bool)
      n387 = case shown="False" w683 {
        tunnel: [w1013 0] -> w652
        frame False {
          w1014 = "?BSI_ReadData"  # ?BSI_ReadData
          n388 = stacked-sequence {
            seq-local: [w1015 _ _] -> [_ _ w1070]
            tunnel: w1014 -> [w1015 _ _]
            tunnel: [_ _ w1048] -> w1013
            frame #0 {
              # "Write Text to Clipboard"
              n389 = String Length(string=w1015) -> (length=w1024:i32)
              n390 = Increment(x=w1024) -> (x+1=w1020:i32)
              n391 = dll-call lib="kernel32" fn="GlobalAlloc"("Flags"=i16 0 ("Format"), "Size"=w1020) -> (w1019:i32)  [unwired: 5 in, 2 out]
              n392 = dll-call lib="kernel32" fn="GlobalLock"("hGlobalMemory"=w1019) -> (w1022:i32)  [unwired: 4 in, 2 out]
              n393 = dll-call lib="kernel32" fn="lstrcpy"("Flags"=w1022, "String"=w1015) -> (w1021:i32)  [unwired: 5 in, 2 out]
              n394 = stacked-sequence {
                tunnel: w1021 -> [_]
                tunnel: w1019 -> [w1043]
                tunnel: [w1042] -> w1018
                frame #0 {
                  n395 = dll-call lib="kernel32" fn="LocalUnlock"("hGlobalMemory"=w1043) -> (w1042:i32)  [unwired: 4 in, 2 out]
                }
              }
              "Error Out 2" <- w1018
              n396 = case shown="0" w1018 {
                selector: w1018 -> [_ w1039]
                tunnel: w1019 -> [w1025 _]
                tunnel: [w1026 w1038] -> w1017
                frame 0 {
                  n397 = dll-call lib="user32" fn="OpenClipboard"("owner"=i16 0) -> (w1027:i32)  [unwired: 4 in, 2 out]
                  n398 = case shown="1, Default" w1027 {
                    selector: w1027 -> [w1031 _]
                    tunnel: [w1029 w1034] -> w1026
                    tunnel: w1025 -> [_ w1033]
                    frame 0 {
                      n399 = Equal To 0?(x=w1031) -> (x = 0?=w1032:bool)
                      n400 = Bundle(w1032, w1031, "source"="Error opening clipboard") -> (w1029:cluster{bool, i32, "source":string})  [unwired: 1 in]
                    }
                    frame 1, Default {
                      n401 = stacked-sequence {
                        tunnel: [_ _ _ cluster{bool, i32, "source":string} {FALSE, 0, "source"=""} ("Output Element")] -> w1034
                        tunnel: w1033 -> [_ w1035 _ _]
                        frame #0 {
                          n402 = dll-call lib="user32" fn="EmptyClipboard"() -> ()  [unwired: 4 in, 2 out]
                        }
                        frame #1 {
                          n403 = dll-call lib="user32" fn="SetClipboardData"("Format"=1, "Data"=w1035) -> ()  [unwired: 6 in, 2 out]
                        }
                        frame #2 {
                          n404 = dll-call lib="user32" fn="CloseClipboard"() -> ()  [unwired: 4 in, 2 out]
                        }
                        frame #3 {
                        }
                      }
                    }
                  }
                }
                frame 1, Default {
                  n405 = Not Equal To 0?(x=w1039) -> (x != 0?=w1040:bool)
                  n406 = Bundle(w1040, w1039, "source"="Error copying text to clipboard") -> (w1038:cluster{bool, i32, "source":string})  [unwired: 1 in]
                }
              }
              "Write error out 2" <- w1017
              n407 = local write "Read Flow Status"("Running" ("Status")) -> ()
            }
            frame #1 {
              # "Wait 500 milliseconds"
              n408 = Wait (ms)(milliseconds to wait=u32 500) -> ()  [unwired: 1 out]
            }
            frame #2 {
              # "Read Text From Clipboard"
              n409 = dll-call lib="user32" fn="OpenClipboard"("owner"=i16 0) -> (w1072:i32)  [unwired: 4 in, 2 out]
              n410 = case shown="1, Default" w1072 {
                selector: w1072 -> [w1078 _]
                tunnel: ["" w1083] -> w1063
                tunnel: [w1076 cluster{bool, i32, "source":string} {FALSE, 0, "source"=""} ("Output Element")] -> w1071
                frame 0 {
                  n411 = Equal To 0?(x=w1078) -> (x = 0?=w1079:bool)
                  n412 = Bundle(w1079, w1078, "source"="No text in clipboard available!") -> (w1076:cluster{bool, i32, "source":string})  [unwired: 1 in]
                }
                frame 1, Default {
                  n413 = dll-call lib="user32" fn="GetClipboardData"("uFormat"=1 ("hGlobalMemory")) -> (w1084:i32)  [unwired: 4 in, 2 out]
                  n414 = dll-call lib="kernel32" fn="GlobalLock"("hGlobalMemory"=w1084) -> (w1083:string, "hGlobalMemory"=w1081:i32)  [unwired: 3 in, 2 out]
                  n415 = stacked-sequence {
                    tunnel: w1081 -> [w1086 _]
                    frame #0 {
                      n416 = dll-call lib="kernel32" fn="LocalUnlock"("hGlobalMemory"=w1086) -> ()  [unwired: 5 in, 2 out]
                    }
                    frame #1 {
                      n417 = dll-call lib="user32" fn="CloseClipboard"() -> ()  [unwired: 4 in, 2 out]
                    }
                  }
                }
              }
              "Text Read From Clipboard 2" <- w1063
              "Read error out 2" <- w1071
              n418 = Search/Split String(string=w1063, search string/char (-)=" ") -> (substring before match=→"First waste string":string, match + rest of string=w1065:string)  [unwired: 1 in, 1 out]
              "Rest of string 1" <- w1065
              n419 = Search/Split String(string=w1065, search string/char (-)=",") -> (substring before match=w1060:string, match + rest of string=w1061:string)  [unwired: 1 in, 1 out]
              n420 = Search/Split String(string=w1061, search string/char (-)="n") -> (substring before match=w1058:string, match + rest of string=w1051:string)  [unwired: 1 in, 1 out]
              "Second Number 2" <- w1058
              "Rest of string 3" <- w1051
              n421 = Equal?(x=w1070, y=w1063) -> (x = y?=w1069:bool)
              n422 = Search/Split String(string=w1051, search string/char (-)="i") -> (substring before match=w1049:string, match + rest of string=w1054:string)  [unwired: 1 in, 1 out]
              "Third Number 3" <- w1049
              "Rest of string 4" <- w1054
              n423 = case shown="True" w1069 {
                tunnel: ["Response OK" "Failed: No Response from Lab Interface"] -> w1068
                frame False {
                }
                frame True {
                }
              }
              "Read Flow Status" <- w1068
              n424 = Search/Split String(string=w1054, search string/char (-)="l") -> (substring before match=w1052:string, match + rest of string=→"Rest of string 5":string)  [unwired: 1 in, 1 out]
              "Fourth Number 3" <- w1052
              n425 = Scan From String(input string=w1060) -> (output 1=w1048:dbl)  [unwired: 4 in, 3 out]
              "Gas Flow 1" <- w1048
              n426 = Scan From String(input string=w1058, initial scan location=1) -> (output 1=→"Gas Flow 2":dbl)  [unwired: 3 in, 3 out]
              n427 = Scan From String(input string=w1049, initial scan location=2) -> (output 1=→"Gas Flow 3":dbl)  [unwired: 3 in, 3 out]
              n428 = Scan From String(input string=w1052, initial scan location=3) -> (output 1=→"Gas Flow 4":dbl)  [unwired: 3 in, 3 out]
            }
          }
        }
        frame True {
        }
      }
      n429 = Merge Signals(w662, w661, w665, w664, w708, w707, w650, w652) -> (w729:dynamicdata)
      n430 = call "Write To Measurement File"("Signals"=w729) -> ()  [unwired: 16 in, 3 out]
      n431 = node-c288() -> ()  [unwired: 1 in, 1 out]
      n432 = Build Array(w739, w738, w737, w736) -> (w731:u32[])
      n433 = Build Array(w732, w735, w734, w733) -> (w730:errorcluster[])
      "loop ind" <- w674
      "Safety Shut Down Temp" <- w713
      "Safety Shut Down Pressure (barg)" <- w696
    }
    n434 = Or(x=w84, y=w92) -> (x .or. y?=w85:bool)
    n435 = case shown="True" w85 {
      frame False {
      }
      frame True {
        w589 = "?BSI_SetFlowSetPoints 0,0,0,0,*,*,*,*,*,*,*,*,*,*,*,*,*,*,*,*,*,*,*,*,*,*,*,*,*,*"  # ?BSI_SetFlowSetPoints 0,0,0,0,*,*,*,*,*,*,*,*,*,*,*,*,*,*,*,*,*,*,*,*,*,*,*,*,*,*
        n436 = stacked-sequence {
          seq-local: [w590 _ _] -> [_ _ w622]
          tunnel: w589 -> [w590 _ _]
          frame #0 {
            # "Write Text to Clipboard"
            n437 = String Length(string=w590) -> (length=w598:i32)
            n438 = Increment(x=w598) -> (x+1=w594:i32)
            n439 = dll-call lib="kernel32" fn="GlobalAlloc"("Flags"=i16 0 ("Format"), "Size"=w594) -> (w593:i32)  [unwired: 5 in, 2 out]
            n440 = dll-call lib="kernel32" fn="GlobalLock"("hGlobalMemory"=w593) -> (w596:i32)  [unwired: 4 in, 2 out]
            n441 = dll-call lib="kernel32" fn="lstrcpy"("Flags"=w596, "String"=w590) -> (w595:i32)  [unwired: 5 in, 2 out]
            n442 = stacked-sequence {
              tunnel: w595 -> [_]
              tunnel: w593 -> [w617]
              tunnel: [w616] -> w592
              frame #0 {
                n443 = dll-call lib="kernel32" fn="LocalUnlock"("hGlobalMemory"=w617) -> (w616:i32)  [unwired: 4 in, 2 out]
              }
            }
            n444 = case shown="0" w592 {
              selector: w592 -> [_ w613]
              tunnel: w593 -> [w599 _]
              tunnel: [w600 w612] -> _
              frame 0 {
                n445 = dll-call lib="user32" fn="OpenClipboard"("owner"=i16 0) -> (w601:i32)  [unwired: 4 in, 2 out]
                n446 = case shown="1, Default" w601 {
                  selector: w601 -> [w605 _]
                  tunnel: [w603 w608] -> w600
                  tunnel: w599 -> [_ w607]
                  tunnel: w599 -> [_ _]
                  frame 0 {
                    n447 = Equal To 0?(x=w605) -> (x = 0?=w606:bool)
                    n448 = Bundle(w606, w605, "source"="Error opening clipboard") -> (w603:cluster{bool, i32, "source":string})  [unwired: 1 in]
                  }
                  frame 1, Default {
                    n449 = stacked-sequence {
                      tunnel: [_ _ _ cluster{bool, i32, "source":string} {FALSE, 0, "source"=""} ("Output Element")] -> w608
                      tunnel: w607 -> [_ w609 _ _]
                      frame #0 {
                        n450 = dll-call lib="user32" fn="EmptyClipboard"() -> ()  [unwired: 4 in, 2 out]
                      }
                      frame #1 {
                        n451 = dll-call lib="user32" fn="SetClipboardData"("Format"=1, "Data"=w609) -> ()  [unwired: 6 in, 2 out]
                      }
                      frame #2 {
                        n452 = dll-call lib="user32" fn="CloseClipboard"() -> ()  [unwired: 4 in, 2 out]
                      }
                      frame #3 {
                      }
                    }
                  }
                }
              }
              frame 1, Default {
                n453 = Not Equal To 0?(x=w613) -> (x != 0?=w614:bool)
                n454 = Bundle(w614, w613, "source"="Error copying text to clipboard") -> (w612:cluster{bool, i32, "source":string})  [unwired: 1 in]
              }
            }
            n455 = local write "Write Set Point Status 2"("Running" ("Status")) -> ()
          }
          frame #1 {
            # "Wait 500 milliseconds"
            n456 = Wait (ms)(milliseconds to wait=u32 500) -> ()  [unwired: 1 out]
          }
          frame #2 {
            # "Read Text From Clipboard"
            n457 = dll-call lib="user32" fn="OpenClipboard"("owner"=i16 0) -> (w623:i32)  [unwired: 4 in, 2 out]
            n458 = case shown="1, Default" w623 {
              selector: w623 -> [w629 _]
              tunnel: ["" w634] -> w619
              tunnel: [w627 cluster{bool, i32, "source":string} {FALSE, 0, "source"=""} ("Output Element")] -> _
              frame 0 {
                n459 = Equal To 0?(x=w629) -> (x = 0?=w630:bool)
                n460 = Bundle(w630, w629, "source"="No text in clipboard available!") -> (w627:cluster{bool, i32, "source":string})  [unwired: 1 in]
              }
              frame 1, Default {
                n461 = dll-call lib="user32" fn="GetClipboardData"("uFormat"=1 ("hGlobalMemory")) -> (w635:i32)  [unwired: 4 in, 2 out]
                n462 = dll-call lib="kernel32" fn="GlobalLock"("hGlobalMemory"=w635) -> (w634:string, "hGlobalMemory"=w632:i32)  [unwired: 3 in, 2 out]
                n463 = stacked-sequence {
                  tunnel: w632 -> [w637 _]
                  frame #0 {
                    n464 = dll-call lib="kernel32" fn="LocalUnlock"("hGlobalMemory"=w637) -> ()  [unwired: 5 in, 2 out]
                  }
                  frame #1 {
                    n465 = dll-call lib="user32" fn="CloseClipboard"() -> ()  [unwired: 4 in, 2 out]
                  }
                }
              }
            }
            "Text Read From Clipboard 5" <- w619
            n466 = Equal?(x=w622, y=w619) -> (x = y?=w621:bool)
            n467 = case shown="True" w621 {
              tunnel: ["Response OK" "Failed: No Response from Lab Interface"] -> w620
              frame False {
              }
              frame True {
              }
            }
            "Write Set Point Status 2" <- w620
          }
        }
      }
    }
    n468 = node-c288(w98) -> ()  [unwired: 1 out]
  }
  n469 = call <vilib>:"DAQmx Stop Task.vi"("task/channels in"=w4, "error in"=w3) -> ("task out"=w6:refnum<k21>, "error out"=w5:errorcluster)  [unwired: 12 in]
  n470 = Index Array(array=w33, index=0) -> (element=w35:u32)
  n471 = Index Array(array=w32, index=0) -> (element=w34:errorcluster)
  n472 = call <vilib>:"DAQmx Clear Task.vi"("task in"=w6, "error in"=w5) -> ()  [unwired: 13 in, 1 out]
  n473 = call "NCS_CloseDevice.vi"("error in (no error)"=w34, "device handle"=w35) -> ()  [unwired: 1 out]
  n474 = call "CN7500_Write Set Point Value.vi"("Target Set Point Value"=25, "error in (no error)"=w21, "Controller Number"=w24, "VISA In"=w20) -> ("error out"=w26:errorcluster, "VISA Out"=w27:refnum<visa-resource-name>)  [unwired: 6 in]
  n475 = call "CN7500_Close.vi"("error in (no error)"=w26, "VISA resource name"=w27) -> ()  [unwired: 9 in, 1 out]
